vi "run.vi"() -> ()   [LabVIEW 2017]
uses:
  <vilib>/Instr/_visa.llb/VISA Configure Serial Port (Instr).vi
panel:
  in  "设备检查":bool
  out "预压？":bool=TRUE
  in  "精度":dbl=0.0005
  out "测试时断开电源？":bool=TRUE
  out "多通道/单通道":bool=TRUE
  out "压力点个数":i32
  in  "退出":bool
  out "组装调试":bool=TRUE
  in  "控制板":refnum<visa-resource-name>="COM16"
  in  "时漂测试间隔时间(min)":i32=30
  in  "时漂测试":bool
  out "时漂":dbl
  out "时漂测试数据":i32[](listbox)
  out "时漂常压输出":string[][](array[string])
  out "错误输出 3":errorcluster caption="错误输出"
  in  "温度显示编号":enum16{""}(ring)
  out "曲线拟合参数":string
  in  "传感器显示编号":u16(ring) items=["1", "2", "3", "4", "5", "6", "7", "8", "9"]
  out "显示数据":i32[](listbox)
  out "XY图":cluster{i32[], i32[]}[](graph)
  out "结束":bool
  out "显示数据":string[][](array[string])
  out "数据":string[][](array[string])
  out "错误输出 2":errorcluster caption="错误输出"
  out "压力稳定":bool
  out "压力最小值":dbl
  out "压力最大值":dbl
  out "保存名":string
  out "path":string
  out "错误输出":errorcluster
  out "恒温结束时间":string
  out "恒温开始时间":string
  out "恒温结束分钟":i32
  out "恒温结束小时":i32
  out "分钟":i32
  out "小时":i32
  out "开始上电":bool
  out "恒温开始":bool
  out "开始采集":bool
  out "传感器预热":bool
  out "恒温中":bool
  out "温度校验次数":dbl
  out "实时压力kPa":string
  out "实时温度℃":dbl
  out "当前设定温度℃":dbl
  out "温度点":i32
  in  "温度（℃）":dbl[](array[numeric])=[25.0]
  in  "CONST820":refnum<visa-resource-name>="COM3"
  in  "传感器顺序编号（从1开始）":string[](array[string])=["1", "2", "3", "4", "5", "6", "7", "8", "9"]
  in  "第二路电流 （A）":dbl=1.0
  in  "第二路电压（V）":dbl=5.0
  in  "第一路电压（V）":dbl=15.0
  in  "第一路电流（A）":dbl=1.0
  in  "DH1766-2":refnum<visa-resource-name>="COM5"
  in  "检定次数":i32=1
  in  "恒温时间（分钟）":i32=60
  in  "传感器预热时间（分钟）":i32=30
  in  "GWS":refnum<visa-resource-name>="COM4"
  in  "温度上限（℃）":dbl=75.0
  in  "温度下限（℃）":dbl=-45.0
  in  "HP34401":refnum<visa-resource-name>="COM1"
  in  "压力设定值（KPa）":dbl[](array[numeric])=[100.0, 15000.0]
  in  "STOP":bool
  out "loging":string
  out "GWS":bool
  in  "START":bool
  # "多通道 传感器测试系统"
  # "注意：\n系统测试与调试被整体集成在一起，可在主界面统一调用该页面。该页面执行完成后，返回主页面进行参数计算。\n温度设置：如需要进行自动 参数计算，请设置20℃附近常温。如不需要请忽略。\n传感器编号请从1开始，逐加。\n如需进行时漂测试，请只设置常温常压。\n\n调试测试时分两步进行：\n1、补偿电阻计算测试：\n温度设置-40℃，70℃。压力设置20KPa,15000KPa.\n2、偏置增益计算测试：\n温度设置20℃。压力设置20KPa, 100KPa, 1000KPa, 5000KPa, 10000KPa, 15000KPa。\n\n系统测试时：\n温度设置20℃， 压力设置20KPa, 100KPa, 1000KPa, 5000KPa, 10000KPa, 15000KPa。\n\n温漂测试时：\n温度设置20℃， 压力设置100KPa"
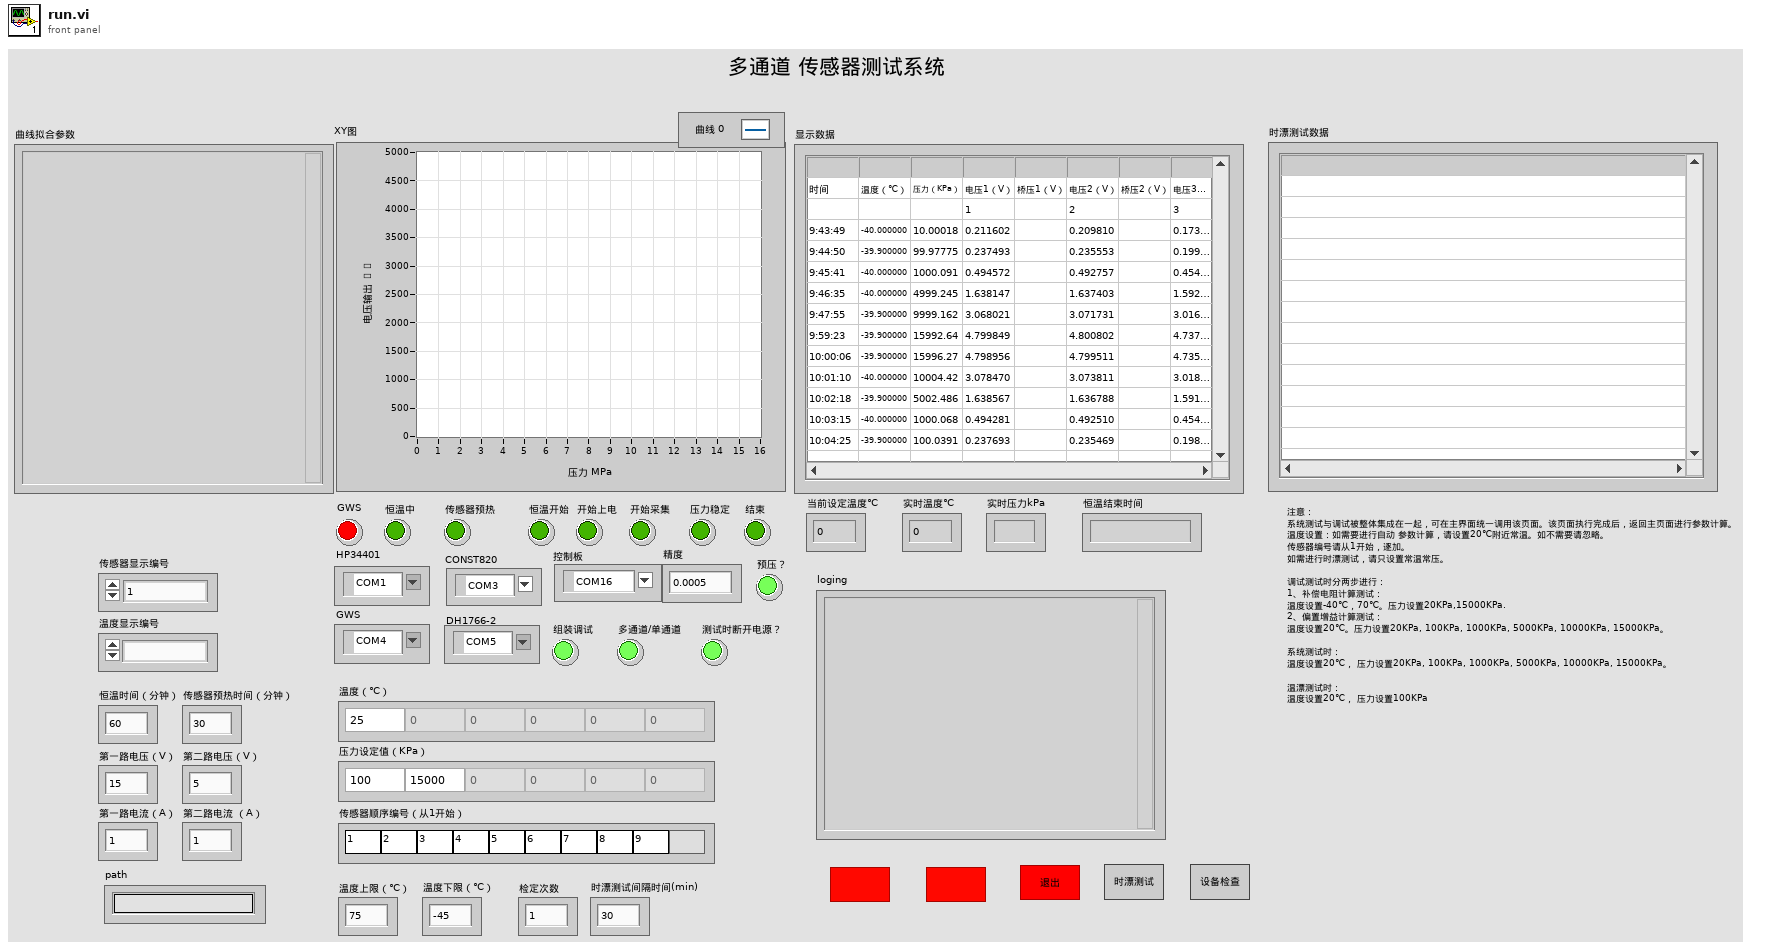
[diagram p1: front panel]
types:
  T1 = enum8{"Enabled", "Disabled", "Disabled and Grayed Out"}
  T2 = enum16{"open", "open or create", "create or replace", "create", "open (read-only)"}
  T3 = enum32{"Invalid", "Standard", "Closed", "Hidden", "Minimized", "Maximized"}
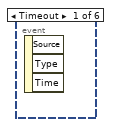
[diagram p2: hidden frame]
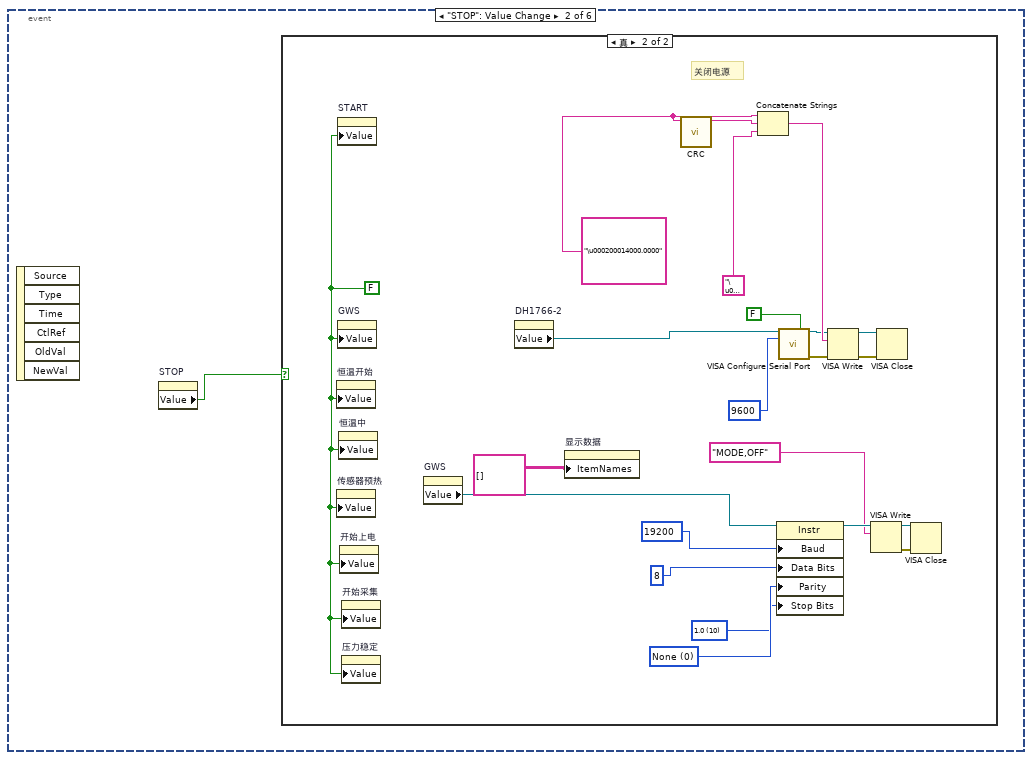
[diagram p3: hidden frame]
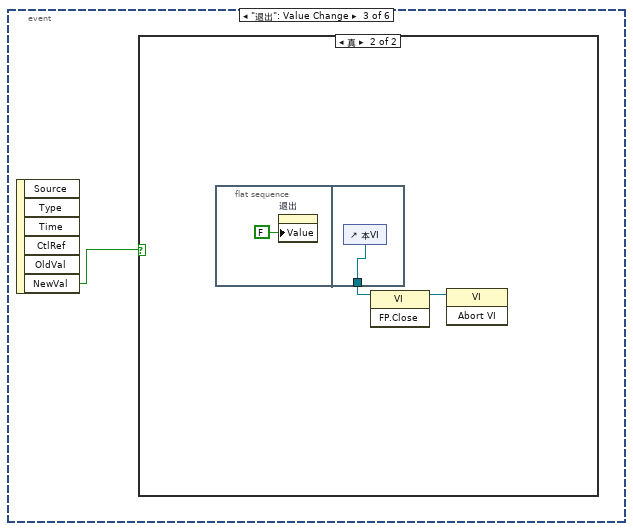
[diagram p5: hidden frame]
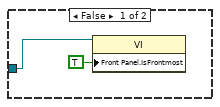
[diagram p8: hidden frame]
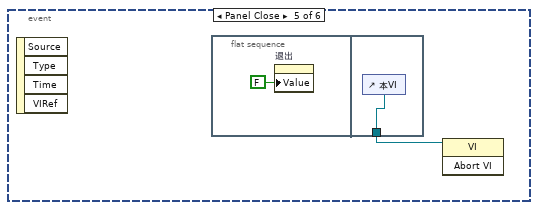
[diagram p9: hidden frame]
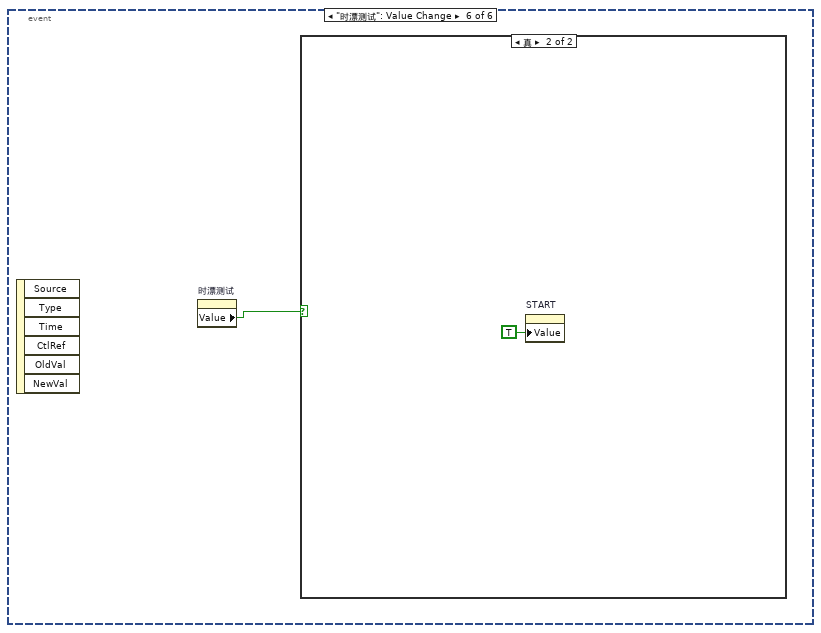
[diagram p10: hidden frame]
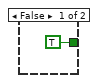
[diagram p14: hidden frame]
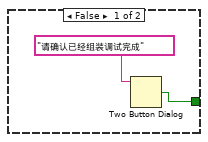
[diagram p15: hidden frame]
diagram:
  n1 = flat-sequence {
    frame #0 {
      w4 = FALSE ("恒温开始")
      w3 = FALSE ("参数计算")
      w5 = string[][] []
      w10 = ""
      w11 = 0.0
      w2 = FALSE
      # "时漂测试开始不用规定"
      n2 = disable-structure shown="禁用" {
        frame Disabled {
          n3 = property on="检定次数" class="DigNum (严格)" props=["Value"]() -> ()  [unwired: 3 in, 2 out]
        }
        frame Enabled {
        }
      }
      n4 = property on="START" class="Bool (严格)"("Value"=w2) -> ()  [unwired: 2 in, 2 out]
      n5 = property on="STOP" class="Bool (严格)"("Value"=w2) -> ()  [unwired: 2 in, 2 out]
      n6 = property on="设备检查" class="Bool (严格)"("Value"=w2) -> ()  [unwired: 2 in, 2 out]
      n7 = property on="显示数据" class="MCListbox (严格)"("ItemNames"=w5) -> ()  [unwired: 2 in, 2 out]
      n8 = property on="时漂测试数据" class="MCListbox (严格)"("ItemNames"=w5) -> ()  [unwired: 2 in, 2 out]
      n9 = property on="时漂测试" class="Bool (严格)"("Value"=w3) -> ()  [unwired: 2 in, 2 out]
      n10 = property on="时漂常压输出" class="Arr (严格)"("Value"=w5) -> ()  [unwired: 2 in, 2 out]
      n11 = property on="退出" class="Bool (严格)"("Value"=w3) -> ()  [unwired: 2 in, 2 out]
      "GWS" <- w2
      "loging" <- w10
      "温度点" <- 0 ("温度点")
      "当前设定温度℃" <- w11
      "实时温度℃" <- w11
      "实时压力kPa" <- w10
      "温度校验次数" <- 5.0 ("温度校验次数")
      "恒温开始" <- w4
      "恒温中" <- w4
      "传感器预热" <- w4
      "恒温结束时间" <- "" ("恒温结束时间")
      "开始上电" <- w4
      "开始采集" <- w4
      "压力稳定" <- w4
      "数据" <- w5
      "显示数据" <- w5
      "结束" <- w2
      "曲线拟合参数" <- "" ("曲线拟合参数")
      "时漂常压输出" <- w5
      "XY图" <- cluster{i32[], i32[]}[] []
    }
    frame #1 {
      n12 = while {
        stop <- FALSE stop-if-true
        # "start循环"
        n13 = property on="START" class="Bool (严格)"() -> ("Value"=w14:bool)  [unwired: 2 in, 2 out]
        n14 = And(x=w14, y=TRUE) -> (x .and. y?=w13:bool)
        n15 = case shown="真" w13 {
          frame False {
          }
          frame True {
            # "start点击判断"
            # "启动系统start"
            n16 = First Call?() -> (First Call?: T/F=w17:bool)
            n17 = property on="传感器预热时间（分钟）" class="DigNum (严格)"() -> ("Value"=w42:i32)  [unwired: 2 in, 2 out]
            n18 = property on="恒温时间（分钟）" class="DigNum (严格)"() -> ("Value"=w43:i32)  [unwired: 2 in, 2 out]
            n19 = property on="温度下限（℃）" class="DigNum (严格)"() -> ("Value"=w58:dbl)  [unwired: 2 in, 2 out]
            n20 = property on="温度上限（℃）" class="DigNum (严格)"() -> ("Value"=w59:dbl)  [unwired: 2 in, 2 out]
            n21 = property on="GWS" class="VISAName"() -> ("Value"=w71:refnum<visa-resource-name>)  [unwired: 2 in, 2 out]
            n22 = property on="检定次数" class="DigNum (严格)"() -> ("Value"=w40:i32)  [unwired: 2 in, 2 out]
            n23 = property on="DH1766-2" class="VISAName"() -> ("Value"=w69:refnum<visa-resource-name>)  [unwired: 2 in, 2 out]
            n24 = property on="CONST820" class="VISAName"() -> ("Value"=w67:refnum<visa-resource-name>)  [unwired: 2 in, 2 out]
            n25 = property on="HP34401" class="VISAName"() -> ("Value"=w65:refnum<visa-resource-name>)  [unwired: 2 in, 2 out]
            n26 = property on="温度（℃）" class="Arr (严格)"() -> ("Value"=w30:dbl[])  [unwired: 2 in, 2 out]
            n27 = property on="压力设定值（KPa）" class="Arr (严格)"() -> ("Value"=w35:dbl[])  [unwired: 2 in, 2 out]
            n28 = property on="传感器顺序编号（从1开始）" class="Arr (严格)"() -> ("Value"=w25:string[])  [unwired: 2 in, 2 out]
            n29 = case shown="真" w17 {
              tunnel: [TRUE ("T button?") w79] -> w16
              frame False {
              }
              frame True {
                n30 = property on="组装调试" class="Bool (严格)"() -> ("Value"=w80:bool)  [unwired: 2 in, 2 out]
                n31 = case shown="真" w80 {
                  tunnel: [w81 w83] -> w79
                  frame False {
                    n32 = Two Button Dialog(message="请确认已经组装调试完成" ("消息")) -> (T button?=w81:bool)  [unwired: 2 in]
                  }
                  frame True {
                    n33 = Two Button Dialog(message="请确认进行组装调试" ("消息")) -> (T button?=w83:bool)  [unwired: 2 in]
                  }
                }
              }
            }
            n34 = Greater Than 0?(x=w40) -> (x > 0?=w39:bool)
            n35 = Greater Than 0?(x=w42) -> (x > 0?=w54:bool)
            n36 = Greater Than 0?(x=w43) -> (x > 0?=w44:bool)
            n37 = Greater Or Equal?(x=w43, y=w42) -> (x >= y?=w41:bool)
            n38 = Array Size(array=w30) -> (size(s)=w29:i32)
            n39 = Array Size(array=w35) -> (size(s)=w33:i32)
            n40 = String Length(string=w71) -> (length=w70:i32)
            n41 = Array Size(array=w25) -> (size(s)=w24:i32)
            n42 = String Length(string=w69) -> (length=w68:i32)
            n43 = String Length(string=w67) -> (length=w66:i32)
            n44 = String Length(string=w65) -> (length=w64:i32)
            n45 = Less Or Equal To 0?(x=w29) -> (x <= 0?=w27:bool)
            n46 = Less Or Equal To 0?(x=w33) -> (x <= 0?=w32:bool)
            n47 = Greater Or Equal?(x=w59, y=w58) -> (x >= y?=w57:bool)
            n48 = Less Or Equal To 0?(x=w24) -> (x <= 0?=w23:bool)
            n49 = Equal?(x=w70, y=0) -> (x = y?=w73:bool)
            n50 = Equal?(x=w68, y=0) -> (x = y?=w72:bool)
            n51 = Equal?(x=w66, y=0) -> (x = y?=w75:bool)
            n52 = Equal?(x=w64, y=0) -> (x = y?=w76:bool)
            n53 = case shown="假" w57 {
              tunnel: ["温度上限>=温度下限 \n" _] -> w51
              frame False {
              }
              frame True {
              }
            }
            n54 = And(x=w44, y=w54) -> (x .and. y?=w38:bool)
            n55 = And(x=w39, y=w38) -> (x .and. y?=w37:bool)
            n56 = And(x=w37, y=w41) -> (x .and. y?=w36:bool)
            n57 = case shown="真" w27 {
              tunnel: [_ "请设置温度\n"] -> w28
              frame False {
              }
              frame True {
              }
            }
            n58 = case shown="真" w32 {
              tunnel: [_ "请设置压力\n"] -> w34
              frame False {
              }
              frame True {
              }
            }
            n59 = case shown="真" w23 {
              tunnel: [_ "请设置传感器编号\n"] -> w21
              frame False {
              }
              frame True {
              }
            }
            n60 = Not(x=w57) -> (.not. x?=w55:bool)
            n61 = Or(x=w72, y=w73) -> (x .or. y?=w74:bool)
            n62 = Or(x=w75, y=w74) -> (x .or. y?=w77:bool)
            n63 = Or(x=w76, y=w77) -> (x .or. y?=w56:bool)
            n64 = Not(x=w36) -> (.not. x?=w52:bool)
            n65 = case shown="假" w36 {
              tunnel: ["检定次数、恒温时间、传感器预热时间均应大于0、恒温时间>=传感器预热时间 " _] -> w47
              frame False {
              }
              frame True {
              }
            }
            n66 = Or(x=w56, y=w55) -> (x .or. y?=w53:bool)
            n67 = case shown="真" w56 {
              tunnel: [_ "部分资源未引用 "] -> w48
              frame False {
              }
              frame True {
              }
            }
            n68 = Not(x=w16) -> (.not. x?=w18:bool)
            n69 = Or(x=w53, y=w52) -> (x .or. y?=w31:bool)
            n70 = Or(x=w31, y=w32) -> (x .or. y?=w26:bool)
            n71 = Or(x=w26, y=w27) -> (x .or. y?=w22:bool)
            n72 = Or(x=w22, y=w23) -> (x .or. y?=w20:bool)
            n73 = Or(x=w20, y=w18) -> (x .or. y?=w19:bool)
            n74 = Concatenate Strings(w48, w51, w47, w34, w28, w21) -> (w45:string)
            n75 = Search and Replace String(input string=w45, search string=" " ("搜索字符串"), replace string="\r") -> (result string=w49:string)  [unwired: 5 in, 3 out]
            n76 = case shown="假" w19 {
              tunnel: w49 -> [_ w950]
              frame False {
                n77 = First Call?() -> (First Call?: T/F=w90:bool)
                n78 = case shown="真" w90 {
                  frame False {
                  }
                  frame True {
                    n79 = property on="传感器顺序编号（从1开始）" class="Arr (严格)"() -> ("Value"=w96:string[])  [unwired: 2 in, 2 out]
                    n80 = property on="时漂测试" class="Bool (严格)"() -> ("Value"=w101:bool)  [unwired: 2 in, 2 out]
                    n81 = disable-structure shown="禁用" {
                      frame Disabled {
                        n82 = property on="温度（℃）" class="Arr (严格)"() -> ("Value"=w107:dbl[])  [unwired: 2 in, 2 out]
                        n83 = Sort 1D Array(array=w107) -> (sorted array=w108:dbl[])
                        n84 = property on="温度（℃）" class="Arr (严格)"("Value"=w108) -> ()  [unwired: 2 in, 2 out]
                      }
                      frame Enabled {
                      }
                    }
                    n85 = property on="压力设定值（KPa）" class="Arr (严格)"() -> ("Value"=w95:dbl[])  [unwired: 2 in, 2 out]
                    n86 = for {
                      tunnel: w96 -> [w118] mode=indexing
                      shift-right: [w120] -> w93
                      shift-left: string[] [] -> [w119]
                      n87 = call <vilib>:"Trim Whitespace.vi"("string"=w118) -> ("trimmed string"=w117:string)  [unwired: 1 in]
                      n88 = String Length(string=w117) -> (length=w122:i32)
                      n89 = Equal To 0?(x=w122) -> (x = 0?=w121:bool)
                      n90 = case shown="真" w121 {
                        tunnel: w117 -> [w125 _]
                        tunnel: [w124 w126] -> w120
                        tunnel: w119 -> [w123 w128]
                        frame False {
                          n91 = Build Array (concatenate)(w123, w125) -> (w124:string[])
                        }
                        frame True {
                          n92 = Insert Into Array(array=w128, new element=string[] []) -> (w126:string[])  [unwired: 1 in]
                        }
                      }
                    }
                    n93 = property on="恒温时间（分钟）" class="DigNum (严格)"() -> ("Value"=w104:i32)  [unwired: 2 in, 2 out]
                    n94 = property on="时漂测试间隔时间(min)" class="DigNum (严格)"() -> ("Value"=w102:i32)  [unwired: 2 in, 2 out]
                    n95 = for {
                      tunnel: w95 -> [w109] mode=indexing
                      shift-right: [w112] -> w94
                      shift-left: dbl[] [] -> [w111]
                      n96 = Less Or Equal To 0?(x=w109) -> (x <= 0?=w110:bool)
                      n97 = case shown="假" w110 {
                        tunnel: [w115 w116] -> w112
                        tunnel: w111 -> [w114 w116]
                        tunnel: w109 -> [w113 _]
                        frame False {
                          n98 = Build Array (concatenate)(w114, w113) -> (w115:dbl[])
                        }
                        frame True {
                        }
                      }
                    }
                    n99 = Multiply(x=w102, y=8) -> (x*y=w103:i32)
                    n100 = Add(x=w103, y=w104) -> (x+y=w105:i32)
                    n101 = Number To Decimal String(number=w105) -> (decimal integer string=w106:string)  [unwired: 1 in]
                    n102 = case shown="真" w101 {
                      tunnel: w106 -> [_ w131]
                      frame False {
                      }
                      frame True {
                        n103 = Concatenate Strings("计算时间漂移、大约用时：" ("字符串"), w131, " min", "\n") -> (w133:string)
                        n104 = property on="loging" class="Str"("Value"=w133) -> ()  [unwired: 2 in, 2 out]
                      }
                    }
                    n105 = property on="压力设定值（KPa）" class="Arr (严格)"("Value"=w94) -> ()  [unwired: 2 in, 2 out]
                    n106 = Array Size(array=w94) -> (size(s)=w97:i32)
                    n107 = property on="传感器顺序编号（从1开始）" class="Arr (严格)"("Value"=w93) -> ()  [unwired: 2 in, 2 out]
                    n108 = property on="检定次数" class="DigNum (严格)"("DisabledEnum"=T1."Enabled" ("禁用")) -> ()  [unwired: 2 in, 2 out]
                    n109 = property on="压力点个数" class="DigNum (严格)"("Value"=w97) -> ()  [unwired: 2 in, 2 out]
                    n110 = property on="结束" class="Bool (严格)"("Value"=FALSE ("结束")) -> ()  [unwired: 2 in, 2 out]
                    n111 = property on="传感器显示编号" class="Ring (严格)"("Strings []"=w93) -> ()  [unwired: 2 in, 2 out]
                  }
                }
                n112 = flat-sequence {
                  frame #0 {
                    # "设置正确"
                    # "启动温箱"
                    n113 = property on="GWS" class="Bool (严格)"() -> ("Value"=w134:bool)  [unwired: 2 in, 2 out]
                    n114 = case shown="假" w134 {
                      frame False {
                        n115 = flat-sequence {
                          tunnel: [w160] -> w140
                          tunnel: [w159] -> w139
                          tunnel: [w183] -> w142
                          tunnel: [w182] -> w141
                          tunnel: w140 -> [w180]
                          tunnel: w139 -> [w179]
                          tunnel: [w199] -> w152
                          tunnel: w142 -> [w199]
                          tunnel: [w198] -> w151
                          tunnel: w141 -> [w198]
                          tunnel: w152 -> [w201]
                          tunnel: w151 -> [w202]
                          tunnel: [w201] -> w150
                          tunnel: [w200] -> w147
                          tunnel: w150 -> [w209]
                          tunnel: [w209] -> w149
                          tunnel: [w208] -> w148
                          tunnel: w147 -> [w208]
                          tunnel: w149 -> [w218]
                          tunnel: w148 -> [w217]
                          tunnel: [w213] -> w145
                          tunnel: [w212] -> w144
                          tunnel: [w222] -> w146
                          tunnel: w145 -> [w222]
                          tunnel: w144 -> [w221]
                          tunnel: [w221] -> w143
                          tunnel: w146 -> [w233]
                          tunnel: w143 -> [w232]
                          tunnel: [w228] -> _
                          frame #0 {
                            w164 = u16 10 items=["1.0"=10, "1.5"=15, "2.0"=20] ("stop bits (10: 1 bit)")
                            n116 = property on="GWS" class="VISAName"() -> ("Value"=w163:refnum<visa-resource-name>)  [unwired: 2 in, 2 out]
                            n117 = property on="loging" class="Str"() -> ("Value"=w156:string)  [unwired: 2 in, 2 out]
                            n118 = Concatenate Strings(w156, "\n启动温箱" ("字符串"), "\n") -> (w155:string)
                            n119 = call-poly "VISA Configure Serial Port"("VISA resource name"=w163, "baud rate (9600)"=u32 19200, "data bits (8)"=u16 8, "parity (0:none)"=enum16{"None", "Odd", "Even", "Mark", "Space"}."None", "stop bits (10: 1 bit)"=w164) -> ("VISA resource name out"=w158:refnum<visa-resource-name>, "error out"=w162:errorcluster)  [unwired: 9 in]
                            n120 = flat-sequence {
                              tunnel: w162 -> [w169]
                              tunnel: [w169] -> w161
                              tunnel: w158 -> [w168]
                              tunnel: [w168] -> w157
                              frame #0 {
                                n121 = Wait (ms)(milliseconds to wait=u32 20 ("等待时间（毫秒）")) -> ()  [unwired: 1 out]
                              }
                            }
                            n122 = property on="loging" class="Str"("Value"=w155) -> ()  [unwired: 2 in, 2 out]
                            n123 = VISA Open(error in (no error)=w161, VISA resource name=w157) -> (VISA resource name=w160:refnum<visa-resource-name>, error out=w159:errorcluster)  [unwired: 3 in]
                          }
                          frame #1 {
                            w187 = i16 1 ("精度(6)")
                            n124 = property on="时漂测试" class="Bool (严格)"() -> ("Value"=w171:bool)  [unwired: 2 in, 2 out]
                            n125 = property on="loging" class="Str"() -> ("Value"=w178:string)  [unwired: 2 in, 2 out]
                            n126 = property on="温度下限（℃）" class="DigNum (严格)"() -> ("Value"=w189:dbl)  [unwired: 2 in, 2 out]
                            n127 = property on="温度上限（℃）" class="DigNum (严格)"() -> ("Value"=w188:dbl)  [unwired: 2 in, 2 out]
                            n128 = case shown="假" w171 {
                              tunnel: [w193 20.0] -> w172
                              frame False {
                                n129 = property on="温度（℃）" class="Arr (严格)"() -> ("Value"=w195:dbl[])  [unwired: 2 in, 2 out]
                                n130 = property on="温度点" class="DigNum (严格)"() -> ("Value"=w194:i32)  [unwired: 2 in, 2 out]
                                n131 = Index Array(array=w195, index=w194) -> (element=w193:dbl)
                                n132 = property on="当前设定温度℃" class="DigNum (严格)"("Value"=w193) -> ()  [unwired: 2 in, 2 out]
                              }
                              frame True {
                              }
                            }
                            n133 = Number To Fractional String(number=w172, precision (6)=i16 2 ("精度(6)")) -> (F-format string=w174:string)  [unwired: 2 in]
                            n134 = Concatenate Strings(w178, "设定温度 " ("字符串"), w174, "\n") -> (w175:string)
                            n135 = Number To Fractional String(number=w172, precision (6)=w187) -> (F-format string=w192:string)  [unwired: 2 in]
                            n136 = Number To Fractional String(number=w188, precision (6)=w187) -> (F-format string=w190:string)  [unwired: 2 in]
                            n137 = Number To Fractional String(number=w189, precision (6)=w187) -> (F-format string=w191:string)  [unwired: 2 in]
                            n138 = property on="loging" class="Str"("Value"=w175) -> ()  [unwired: 2 in, 2 out]
                            n139 = Concatenate Strings("TEMP,S" ("字符串"), w192, " H" ("字符串"), w190, " L" ("字符串"), w191) -> (w181:string)
                            n140 = VISA Write(VISA resource name=w180, write buffer=w181, error in (no error)=w179) -> (VISA resource name out=w183:refnum<visa-resource-name>, error out=w182:errorcluster)  [unwired: 1 out]
                          }
                          frame #2 {
                            n141 = Wait (ms)(milliseconds to wait=u32 100 ("等待时间（毫秒）")) -> ()  [unwired: 1 out]
                          }
                          frame #3 {
                            n142 = Get Date/Time In Seconds() -> (seconds since 1Jan1904=w205:timestamp)
                            n143 = Get Date/Time String(seconds (now)=w205, want seconds? (F)=TRUE ("需要秒？(F)")) -> (time string=w207:string)  [unwired: 1 in, 1 out]
                            n144 = Concatenate Strings("TIME, " ("字符串"), w207) -> (w203:string)
                            n145 = VISA Write(VISA resource name=w201, write buffer=w203, error in (no error)=w202) -> (error out=w200:errorcluster)  [unwired: 2 out]
                          }
                          frame #4 {
                            n146 = Wait (ms)(milliseconds to wait=u32 100 ("等待时间（毫秒）")) -> ()  [unwired: 1 out]
                          }
                          frame #5 {
                            n147 = VISA Write(VISA resource name=w218, write buffer="TEMP？" ("写入缓冲区"), error in (no error)=w217) -> (VISA resource name out=w219:refnum<visa-resource-name>, error out=w214:errorcluster)  [unwired: 1 out]
                            n148 = property class="Instr"(reference=w219, error in=w214) -> (reference out=w216:refnum<visa-resource-name>, error out=w211:errorcluster, "Bytes at Port"=w215:u32)
                            n149 = VISA Read(VISA resource name=w216, byte count=w215, error in (no error)=w211) -> (VISA resource name out=w213:refnum<visa-resource-name>, error out=w212:errorcluster)  [unwired: 2 out]
                          }
                          frame #6 {
                            n150 = Wait (ms)(milliseconds to wait=u32 100 ("等待时间（毫秒）")) -> ()  [unwired: 1 out]
                          }
                          frame #7 {
                            n151 = property on="loging" class="Str"() -> ("Value"=w227:string)  [unwired: 2 in, 2 out]
                            n152 = Concatenate Strings(w227, "温箱已启动" ("字符串"), "\n") -> (w225:string)
                            n153 = property on="GWS" class="Bool (严格)"("Value"=TRUE ("GWS")) -> ()  [unwired: 2 in, 2 out]
                            n154 = VISA Write(VISA resource name=w233, write buffer="MODE,CONSTANT" ("写入缓冲区"), error in (no error)=w232) -> (VISA resource name out=w230:refnum<visa-resource-name>, error out=w229:errorcluster)  [unwired: 1 out]
                            n155 = property on="loging" class="Str"("Value"=w225) -> ()  [unwired: 2 in, 2 out]
                            n156 = VISA Close(VISA resource name=w230, error in (no error)=w229) -> (error out=w228:errorcluster)
                          }
                        }
                      }
                      frame True {
                      }
                    }
                    n157 = disable-structure shown="禁用" {
                      frame Disabled {
                        n158 = property on="loging" class="Str"() -> ("Value"=w137:string)  [unwired: 2 in, 2 out]
                        n159 = Concatenate Strings(w137, "温箱已启动" ("字符串"), "\n") -> (w138:string)
                        n160 = property on="loging" class="Str"("Value"=w138) -> ()  [unwired: 2 in, 2 out]
                      }
                      frame Enabled {
                      }
                    }
                  }
                  frame #1 {
                    # "温箱温度检查"
                    n161 = property on="温度校验次数" class="DigNum (严格)"() -> ("Value"=w236:dbl)  [unwired: 2 in, 2 out]
                    n162 = disable-structure shown="禁用" {
                      frame Disabled {
                        n163 = property on="温度校验次数" class="DigNum (严格)"() -> ("Value"=w238:dbl)  [unwired: 2 in, 2 out]
                        n164 = Greater Than 0?(x=w238) -> (x > 0?=w237:bool)
                        n165 = case shown="真" w237 {
                          frame False {
                          }
                          frame True {
                            n166 = property on="loging" class="Str"() -> ("Value"=w241:string)  [unwired: 2 in, 2 out]
                            n167 = Concatenate Strings(w241, "温箱温度监控" ("字符串"), "\n") -> (w242:string)
                            n168 = property on="loging" class="Str"("Value"=w242) -> ()  [unwired: 2 in, 2 out]
                          }
                        }
                      }
                      frame Enabled {
                      }
                    }
                    n169 = Greater Than 0?(x=w236) -> (x > 0?=w235:bool)
                    n170 = case shown="真" w235 {
                      frame False {
                      }
                      frame True {
                        n171 = while {
                          stop <- w247 stop-if-true
                          n172 = flat-sequence {
                            tunnel: [w254] -> w252
                            tunnel: [w253] -> w251
                            tunnel: [w261] -> w250
                            tunnel: w252 -> [w261]
                            tunnel: [w260] -> w249
                            tunnel: w251 -> [w260]
                            tunnel: w250 -> [w271]
                            tunnel: w249 -> [w270]
                            frame #0 {
                              n173 = property on="GWS" class="VISAName"() -> (error out=w258:errorcluster, "Value"=w259:refnum<visa-resource-name>)  [unwired: 2 in, 1 out]
                              n174 = VISA Flush I/O Buffer(VISA resource name=w259, error in (no error)=w258) -> (VISA resource name out=w256:refnum<visa-resource-name>, error out=w257:errorcluster)  [unwired: 1 in]
                              n175 = VISA Write(VISA resource name=w256, write buffer="TEMP?" ("写入缓冲区"), error in (no error)=w257) -> (VISA resource name out=w254:refnum<visa-resource-name>, error out=w253:errorcluster)  [unwired: 1 out]
                            }
                            frame #1 {
                              n176 = Wait (ms)(milliseconds to wait=u32 100 ("等待时间（毫秒）")) -> ()  [unwired: 1 out]
                            }
                            frame #2 {
                              n177 = property class="Instr"(reference=w271, error in=w270) -> (reference out=w269:refnum<visa-resource-name>, error out=w267:errorcluster, "Bytes at Port"=w268:u32)
                              n178 = VISA Read(VISA resource name=w269, byte count=w268, error in (no error)=w267) -> (read buffer=w264:string)  [unwired: 3 out]
                              n179 = Match Pattern(string=w264, regular expression="," ("正则表达式")) -> (before substring=w263:string)  [unwired: 1 in, 3 out]
                              n180 = Fract/Exp String To Number(string=w263) -> (number=w266:dbl)  [unwired: 3 in, 1 out]
                              n181 = property on="实时温度℃" class="DigNum (严格)"("Value"=w266) -> ()  [unwired: 2 in, 2 out]
                            }
                            frame #3 {
                              n182 = Wait (ms)(milliseconds to wait=u32 100 ("等待时间（毫秒）")) -> ()  [unwired: 1 out]
                            }
                            frame #4 {
                              w279 = 0.1 ("y")
                              n183 = property on="当前设定温度℃" class="DigNum (严格)"() -> ("Value"=w280:dbl)  [unwired: 2 in, 2 out]
                              n184 = property on="实时温度℃" class="DigNum (严格)"() -> ("Value"=w275:dbl)  [unwired: 2 in, 2 out]
                              n185 = Add(x=w280, y=w279) -> (x+y=w274:dbl)
                              n186 = Greater Or Equal?(x=w274, y=w275) -> (x >= y?=w278:bool)
                              n187 = Subtract(x=w280, y=w279) -> (x-y=w273:dbl)
                              n188 = Greater Or Equal?(x=w275, y=w273) -> (x >= y?=w277:bool)
                              n189 = And(x=w278, y=w277) -> (x .and. y?=w276:bool)
                              n190 = In Range and Coerce(upper limit=w274, x=w275, lower limit=w273) -> ()  [unwired: 2 out]
                              n191 = case shown="真" w276 {
                                frame False {
                                }
                                frame True {
                                n192 = property on="温度校验次数" class="DigNum (严格)"() -> ("Value"=w281:dbl)  [unwired: 2 in, 2 out]
                                n193 = Less Or Equal To 0?(x=w281) -> (x <= 0?=w282:bool)
                                n194 = Decrement(x=w281) -> (x-1=w283:dbl)
                                n195 = case shown="真" w282 {
                                frame False {
                                }
                                frame True {
                                n196 = property on="恒温开始" class="Bool (严格)"("Value"=TRUE ("恒温开始")) -> ()  [unwired: 2 in, 2 out]
                                }
                                }
                                n197 = property on="温度校验次数" class="DigNum (严格)"("Value"=w283) -> ()  [unwired: 2 in, 2 out]
                                }
                              }
                            }
                          }
                          n198 = property on="温度校验次数" class="DigNum (严格)"() -> ("Value"=w248:dbl)  [unwired: 2 in, 2 out]
                          n199 = Less Or Equal To 0?(x=w248) -> (x <= 0?=w247:bool)
                        }
                        n200 = property on="loging" class="Str"() -> ("Value"=w246:string)  [unwired: 2 in, 2 out]
                        n201 = Concatenate Strings(w246, "温箱温度监控、恒温检查中" ("字符串"), "\n") -> (w244:string)
                        n202 = property on="loging" class="Str"("Value"=w244) -> ()  [unwired: 2 in, 2 out]
                      }
                    }
                  }
                  frame #2 {
                    # "恒温到达时间计算"
                    n203 = property on="恒温开始" class="Bool (严格)"() -> ("Value"=w285:bool)  [unwired: 2 in, 2 out]
                    n204 = case shown="真" w285 {
                      frame False {
                      }
                      frame True {
                        w295 = TRUE ("恒温中")
                        n205 = Get Date/Time In Seconds() -> (seconds since 1Jan1904=w309:timestamp)
                        n206 = property on="loging" class="Str"() -> ("Value"=w293:string)  [unwired: 2 in, 2 out]
                        n207 = Get Date/Time String(seconds (now)=w309) -> (date string=w288:string, time string=w286:string)  [unwired: 2 in]
                        n208 = property on="恒温中" class="Bool (严格)"("Value"=w295) -> ()  [unwired: 2 in, 2 out]
                        n209 = Concatenate Strings(w293, "开始恒温，计算恒温时间" ("字符串"), "\n") -> (w290:string)
                        n210 = Concatenate Strings(w288, " " ("字符串"), w286) -> (w289:string)
                        n211 = Match Pattern(string=w286, regular expression=":" ("正则表达式")) -> (before substring=w308:string, after substring=w307:string)  [unwired: 1 in, 2 out]
                        n212 = property on="恒温开始时间" class="Str"("Value"=w289) -> ()  [unwired: 2 in, 2 out]
                        n213 = property on="loging" class="Str"("Value"=w290) -> ()  [unwired: 2 in, 2 out]
                        n214 = property on="恒温开始" class="Bool (严格)"("Value"=FALSE ("恒温开始")) -> ()  [unwired: 2 in, 2 out]
                        n215 = property on="传感器预热" class="Bool (严格)"("Value"=w295) -> ()  [unwired: 2 in, 2 out]
                        n216 = Decimal String To Number(string=w308) -> (number=w301:i32)  [unwired: 2 in, 1 out]
                        n217 = Decimal String To Number(string=w307) -> (number=w300:i32)  [unwired: 2 in, 1 out]
                        n218 = property on="分钟" class="DigNum (严格)"("Value"=w300) -> ()  [unwired: 2 in, 2 out]
                        n219 = property on="小时" class="DigNum (严格)"("Value"=w301) -> ()  [unwired: 2 in, 2 out]
                        n220 = property on="恒温时间（分钟）" class="DigNum (严格)"() -> ("Value"=w299:i32)  [unwired: 2 in, 2 out]
                        n221 = call "cal_end_time.vi"("恒温时间"=w299, "分钟"=w300, "小时"=w301) -> ("结束分钟"=w297:i32, "结束小时"=w298:i32)  [unwired: 7 in]
                        n222 = Number To Decimal String(number=w298, width (-)=i16 2 ("宽度(-)")) -> (decimal integer string=w304:string)
                        n223 = Number To Decimal String(number=w297) -> (decimal integer string=w303:string)  [unwired: 1 in]
                        n224 = Concatenate Strings(w304, ":", w303) -> (w296:string)
                        n225 = property on="恒温结束小时" class="DigNum (严格)"("Value"=w298) -> ()  [unwired: 2 in, 2 out]
                        n226 = property on="恒温结束分钟" class="DigNum (严格)"("Value"=w297) -> ()  [unwired: 2 in, 2 out]
                        n227 = property on="恒温结束时间" class="Str"("Value"=w296) -> ()  [unwired: 2 in, 2 out]
                      }
                    }
                  }
                  frame #3 {
                    # "恒温时间到达"
                    n228 = property on="恒温中" class="Bool (严格)"() -> ("Value"=w311:bool)  [unwired: 2 in, 2 out]
                    n229 = property on="传感器预热" class="Bool (严格)"() -> ("Value"=w310:bool)  [unwired: 2 in, 2 out]
                    n230 = disable-structure shown="禁用" {
                      frame Disabled {
                        n231 = property on="loging" class="Str"() -> ("Value"=w314:string)  [unwired: 2 in, 2 out]
                        n232 = Concatenate Strings(w314, "传感器预热" ("字符串"), "\n") -> (w315:string)
                        n233 = property on="loging" class="Str"("Value"=w315) -> ()  [unwired: 2 in, 2 out]
                      }
                      frame Enabled {
                      }
                    }
                    n234 = case shown="真" w311 {
                      frame False {
                      }
                      frame True {
                        n235 = Get Date/Time In Seconds() -> (seconds since 1Jan1904=w346:timestamp)
                        n236 = Get Date/Time String(seconds (now)=w346) -> (time string=w342:string)  [unwired: 2 in, 1 out]
                        n237 = property on="恒温结束分钟" class="DigNum (严格)"() -> ("Value"=w340:i32)  [unwired: 2 in, 2 out]
                        n238 = property on="恒温结束小时" class="DigNum (严格)"() -> ("Value"=w338:i32)  [unwired: 2 in, 2 out]
                        n239 = Match Pattern(string=w342, regular expression=":" ("正则表达式")) -> (before substring=w345:string, after substring=w344:string)  [unwired: 1 in, 2 out]
                        n240 = Decimal String To Number(string=w345) -> (number=w339:i32)  [unwired: 2 in, 1 out]
                        n241 = Decimal String To Number(string=w344) -> (number=w341:i32)  [unwired: 2 in, 1 out]
                        n242 = Equal?(x=w341, y=w340) -> (x = y?=w337:bool)
                        n243 = Equal?(x=w339, y=w338) -> (x = y?=w336:bool)
                        n244 = And(x=w337, y=w336) -> (x .and. y?=w335:bool)
                        n245 = case shown="真" w335 {
                          frame False {
                          }
                          frame True {
                            n246 = property on="loging" class="Str"() -> ("Value"=w351:string)  [unwired: 2 in, 2 out]
                            n247 = property on="开始采集" class="Bool (严格)"("Value"=TRUE ("开始采集")) -> ()  [unwired: 2 in, 2 out]
                            n248 = property on="恒温中" class="Bool (严格)"("Value"=FALSE ("恒温中")) -> ()  [unwired: 2 in, 2 out]
                            n249 = Concatenate Strings(w351, "恒温时间到" ("字符串"), "\n") -> (w348:string)
                            n250 = property on="loging" class="Str"("Value"=w348) -> ()  [unwired: 2 in, 2 out]
                          }
                        }
                      }
                    }
                    n251 = case shown="真" w310 {
                      frame False {
                      }
                      frame True {
                        n252 = property on="恒温时间（分钟）" class="DigNum (严格)"() -> ("Value"=w332:i32)  [unwired: 2 in, 2 out]
                        n253 = property on="传感器预热时间（分钟）" class="DigNum (严格)"() -> ("Value"=w331:i32)  [unwired: 2 in, 2 out]
                        n254 = property on="分钟" class="DigNum (严格)"() -> ("Value"=w329:i32)  [unwired: 2 in, 2 out]
                        n255 = property on="小时" class="DigNum (严格)"() -> ("Value"=w330:i32)  [unwired: 2 in, 2 out]
                        n256 = Get Date/Time In Seconds() -> (seconds since 1Jan1904=w327:timestamp)
                        n257 = Get Date/Time String(seconds (now)=w327) -> (time string=w323:string)  [unwired: 2 in, 1 out]
                        n258 = Subtract(x=w332, y=w331) -> (x-y=w328:i32)
                        n259 = call "cal_end_time.vi"("恒温时间"=w328, "分钟"=w329, "小时"=w330) -> ("结束分钟"=w319:i32, "结束小时"=w321:i32)  [unwired: 7 in]
                        n260 = Match Pattern(string=w323, regular expression=":" ("正则表达式")) -> (before substring=w326:string, after substring=w325:string)  [unwired: 1 in, 2 out]
                        n261 = Decimal String To Number(string=w326) -> (number=w322:i32)  [unwired: 2 in, 1 out]
                        n262 = Decimal String To Number(string=w325) -> (number=w320:i32)  [unwired: 2 in, 1 out]
                        n263 = Equal?(x=w320, y=w319) -> (x = y?=w317:bool)
                        n264 = Equal?(x=w322, y=w321) -> (x = y?=w318:bool)
                        n265 = And(x=w318, y=w317) -> (x .and. y?=w316:bool)
                        n266 = case shown="真" w316 {
                          frame False {
                          }
                          frame True {
                            n267 = property on="传感器预热" class="Bool (严格)"("Value"=FALSE ("传感器预热")) -> ()  [unwired: 2 in, 2 out]
                            n268 = property on="开始上电" class="Bool (严格)"("Value"=TRUE ("开始上电")) -> ()  [unwired: 2 in, 2 out]
                          }
                        }
                      }
                    }
                  }
                  frame #4 {
                    # "开始 设置电源的两路输出端"
                    n269 = property on="开始上电" class="Bool (严格)"() -> ("Value"=w353:bool)  [unwired: 2 in, 2 out]
                    n270 = case shown="真" w353 {
                      frame False {
                      }
                      frame True {
                        n271 = flat-sequence {
                          tunnel: [w365] -> w359
                          tunnel: [w364] -> w358
                          tunnel: w359 -> [w391]
                          tunnel: [w391] -> w357
                          tunnel: w358 -> [w390]
                          tunnel: [w389] -> w355
                          tunnel: w357 -> [w427]
                          tunnel: [w427] -> w356
                          tunnel: w355 -> [w426]
                          tunnel: [w426] -> w354
                          tunnel: w356 -> [w434]
                          tunnel: w354 -> [w433]
                          frame #0 {
                            # "查询设备是否开启的指令"
                            n272 = while {
                              tunnel: [w368] -> w365
                              tunnel: [w367] -> w364
                              stop <- w369 continue-if-true
                              n273 = property on="DH1766-2" class="VISAName"() -> ("Value"=w384:refnum<visa-resource-name>)  [unwired: 2 in, 2 out]
                              n274 = call-poly "VISA Configure Serial Port"("VISA resource name"=w384) -> ("VISA resource name out"=w381:refnum<visa-resource-name>, "error out"=w379:errorcluster)  [unwired: 13 in]
                              n275 = Concatenate Strings("\u000200018\u0004û" ("字符串"), "\u0003" ("字符串")) -> (w380:string)
                              n276 = VISA Write(VISA resource name=w381, write buffer=w380, error in (no error)=w379) -> (VISA resource name out=w378:refnum<visa-resource-name>, error out=w376:errorcluster)  [unwired: 1 out]
                              n277 = flat-sequence {
                                tunnel: w378 -> [w387]
                                tunnel: [w387] -> w377
                                tunnel: w376 -> [w386]
                                tunnel: [w386] -> w375
                                frame #0 {
                                n278 = Wait (ms)(milliseconds to wait=u32 100 ("等待时间（毫秒）")) -> ()  [unwired: 1 out]
                                }
                              }
                              n279 = property class="Instr"(reference=w377, error in=w375) -> (reference out=w372:refnum<visa-resource-name>, error out=w374:errorcluster, "Bytes at Port"=w373:u32)
                              n280 = VISA Read(VISA resource name=w372, byte count=w373, error in (no error)=w374) -> (VISA resource name out=w368:refnum<visa-resource-name>, read buffer=w371:string, error out=w367:errorcluster)  [unwired: 1 out]
                              n281 = Wait Until Next ms Multiple(millisecond multiple=u32 10 ("毫秒倍数")) -> ()  [unwired: 1 out]
                              n282 = Equal?(x=w371, y="") -> (x = y?=w369:bool)
                              n283 = case shown="真" w369 {
                                frame False {
                                }
                                frame True {
                                n284 = One Button Dialog(message="DH1766电源未开启" ("消息")) -> ()  [unwired: 1 in, 1 out]
                                }
                              }
                            }
                            n285 = property on="loging" class="Str"() -> ("Value"=w363:string)  [unwired: 2 in, 2 out]
                            n286 = Concatenate Strings(w363, "电源输出，开始上电，预热传感器" ("字符串"), "\n") -> (w360:string)
                            n287 = property on="loging" class="Str"("Value"=w360) -> ()  [unwired: 2 in, 2 out]
                          }
                          frame #1 {
                            # "顺序指令执行"
                            n288 = property on="第一路电流（A）" class="DigNum (严格)"() -> ("Value"=w398:dbl)  [unwired: 2 in, 2 out]
                            n289 = property on="第一路电压（V）" class="DigNum (严格)"() -> ("Value"=w397:dbl)  [unwired: 2 in, 2 out]
                            n290 = property on="第二路电压（V）" class="DigNum (严格)"() -> ("Value"=w395:dbl)  [unwired: 2 in, 2 out]
                            n291 = property on="第二路电流 （A）" class="DigNum (严格)"() -> ("Value"=w396:dbl)  [unwired: 2 in, 2 out]
                            n292 = Build Array(w398, w397, w396, w395) -> (w393:dbl[])
                            n293 = Array Size(array=w393) -> (size(s)=w394:i32)
                            n294 = Build Array("\u0002000000", "\u0002000010", "\u0002010000", "\u0002010010") -> (w392:string[])
                            n295 = for {
                              N: w394 -> [_]
                              tunnel: w393 -> [w407] mode=indexing
                              tunnel: w392 -> [w406] mode=indexing
                              tunnel: w391 -> [w405]
                              shift-right: [w403] -> w389
                              shift-left: w390 -> [w404]
                              n296 = flat-sequence {
                                tunnel: w407 -> [w412]
                                tunnel: w406 -> [w411]
                                tunnel: w405 -> [w410]
                                tunnel: w404 -> [w409]
                                tunnel: [w408] -> w403
                                frame #0 {
                                n297 = Number To Fractional String(number=w412, width (-)=7, precision (6)=i16 4 ("精度(6)")) -> (F-format string=w421:string)  [unwired: 1 in]
                                n298 = Search and Replace String(input string=w421, search string=" " ("搜索字符串"), replace string="0" ("子字符串(\"\")"), offset=0 ("偏移量(0)")) -> (result string=w422:string)  [unwired: 4 in, 3 out]
                                n299 = Concatenate Strings(w411, w422) -> (w416:string)
                                n300 = call "CRC.vi"("命令字符串"=w416) -> ("校验字符串"=w415:string)  [unwired: 10 in]
                                n301 = Concatenate Strings(w416, w415, "\u0003" ("字符串")) -> (w414:string)
                                n302 = VISA Write(VISA resource name=w410, write buffer=w414, error in (no error)=w409) -> (error out=w408:errorcluster)  [unwired: 2 out]
                                }
                                frame #1 {
                                n303 = Wait (ms)(milliseconds to wait=u32 100 ("等待时间（毫秒）")) -> ()  [unwired: 1 out]
                                }
                              }
                            }
                          }
                          frame #2 {
                            # "启动所有的节点预热"
                            n304 = property on="多通道/单通道" class="Bool (严格)"() -> ("Value"=w425:bool)  [unwired: 2 in, 2 out]
                            n305 = case shown="真" w425 {
                              frame False {
                              }
                              frame True {
                                n306 = property on="控制板" class="VISAName"() -> ("Value"=w430:refnum<visa-resource-name>)  [unwired: 2 in, 2 out]
                                n307 = property on="传感器顺序编号（从1开始）" class="Arr (严格)"() -> ("Value"=w429:string[])  [unwired: 2 in, 2 out]
                                n308 = Array Size(array=w429) -> (size(s)=w428:i32)
                                n309 = call "prepare_elec_sensor.vi"("传感器数目"=w428, "VISA资源名称"=w430) -> ()  [unwired: 10 in]
                              }
                            }
                          }
                          frame #3 {
                            w437 = "\u000200014111.0000"
                            # "结束配置"
                            n310 = property on="开始上电" class="Bool (严格)"("Value"=FALSE ("开始上电")) -> ()  [unwired: 2 in, 2 out]
                            n311 = call "CRC.vi"("命令字符串"=w437) -> ("校验字符串"=w438:string)  [unwired: 10 in]
                            n312 = Concatenate Strings(w437, w438, "\u0003" ("字符串")) -> (w439:string)
                            n313 = VISA Write(VISA resource name=w434, write buffer=w439, error in (no error)=w433) -> (VISA resource name out=w436:refnum<visa-resource-name>, error out=w435:errorcluster)  [unwired: 1 out]
                            n314 = VISA Close(VISA resource name=w436, error in (no error)=w435) -> (error out=→"错误输出":errorcluster)
                          }
                        }
                      }
                    }
                  }
                  frame #5 {
                    # "数值有效判断"
                    # "开始采集数据"
                    n315 = property on="开始采集" class="Bool (严格)"() -> ("Value"=w441:bool)  [unwired: 2 in, 2 out]
                    n316 = case shown="真" w441 {
                      frame False {
                      }
                      frame True {
                        n317 = flat-sequence {
                          tunnel: [w477] -> w442
                          frame #0 {
                            n318 = property on="预压？" class="Bool (严格)"() -> ("Value"=w474:bool)  [unwired: 2 in, 2 out]
                            n319 = case shown="真" w474 {
                              frame False {
                              }
                              frame True {
                                n320 = property on="压力设定值（KPa）" class="Arr (严格)"() -> ("Value"=w475:dbl[])  [unwired: 2 in, 2 out]
                                n321 = property on="CONST820" class="VISAName"() -> ("Value"=w476:refnum<visa-resource-name>)  [unwired: 2 in, 2 out]
                                n322 = call "prepare_press.vi"("压力设定值（KPa）"=w475, "CONST820"=w476) -> ()  [unwired: 10 in]
                              }
                            }
                          }
                          frame #1 {
                            n323 = property on="时漂测试" class="Bool (严格)"() -> ("Value"=w477:bool)  [unwired: 2 in, 2 out]
                          }
                        }
                        n324 = Get Date/Time String() -> (date string=w465:string, time string=w453:string)  [unwired: 3 in]
                        n325 = Search and Replace String(input string=w465, search string="/" ("搜索字符串"), replace string="" ("替换字符串(\"\")")) -> (result string=w471:string)  [unwired: 5 in, 3 out]
                        n326 = Search and Replace String(input string=w453, search string=":" ("搜索字符串"), replace string="" ("替换字符串(\"\")")) -> (result string=w457:string)  [unwired: 5 in, 3 out]
                        n327 = property on="loging" class="Str"() -> ("Value"=w463:string)  [unwired: 2 in, 2 out]
                        n328 = Search and Replace String(input string=w471, search string="/" ("搜索字符串"), replace string="" ("替换字符串(\"\")")) -> (result string=w468:string)  [unwired: 5 in, 3 out]
                        n329 = Concatenate Strings(w463, "恒温变压数据采集中" ("字符串"), "\n") -> (w460:string)
                        n330 = Search and Replace String(input string=w457, search string=":" ("搜索字符串"), replace string="" ("替换字符串(\"\")")) -> (result string=w452:string)  [unwired: 5 in, 3 out]
                        n331 = Concatenate Strings(w468, "" ("字符串")) -> (w466:string)
                        n332 = property on="loging" class="Str"("Value"=w460) -> ()  [unwired: 2 in, 2 out]
                        n333 = Concatenate Strings(w466, "_" ("字符串"), w452) -> (w449:string)
                        "保存名" <- w449
                        n334 = property on="当前设定温度℃" class="DigNum (严格)"() -> ("Value"=w464:dbl)  [unwired: 2 in, 2 out]
                        n335 = Number To Fractional String(number=w464, precision (6)=i16 1 ("精度(6)")) -> (F-format string=w447:string)  [unwired: 2 in]
                        n336 = Search and Replace String(input string=w447, search string="." ("搜索字符串"), replace string="" ("替换字符串(\"\")")) -> (result string=w444:string)  [unwired: 5 in, 3 out]
                        n337 = Concatenate Strings(w449, "_" ("字符串"), w444) -> (→"path":string)
                        n338 = case shown="真" w442 {
                          frame False {
                          }
                          frame True {
                            # "时漂执行序列"
                            # "时间漂移测试"
                            n339 = flat-sequence {
                              frame #0 {
                                n340 = for {
                                N: 9 -> [_]
                                i -> [w684]
                                # "执行序列"
                                n341 = flat-sequence {
                                tunnel: [w700] -> w695
                                tunnel: [w699] -> w689
                                tunnel: [w697] -> w685
                                tunnel: [w704] -> w696
                                tunnel: w695 -> [w704]
                                tunnel: [w703] -> w694
                                tunnel: w689 -> [w703]
                                tunnel: [w701] -> w686
                                tunnel: w685 -> [w701]
                                tunnel: w696 -> [w710]
                                tunnel: w694 -> [w709]
                                tunnel: [w708] -> w693
                                tunnel: [w707] -> w692
                                tunnel: [w706] -> w688
                                tunnel: [w705] -> w687
                                tunnel: w686 -> [w705]
                                tunnel: w693 -> [w724]
                                tunnel: w692 -> [w723]
                                tunnel: [w722] -> w691
                                tunnel: [w721] -> w690
                                tunnel: w688 -> [w720]
                                tunnel: w687 -> [w719]
                                tunnel: w691 -> [w750]
                                tunnel: w690 -> [w749]
                                tunnel: w684 -> [w838]
                                frame #0 {
                                w697 = 100.0 ("设定")
                                # "压力固定值"
                                n342 = property on="CONST820" class="VISAName"() -> ("Value"=w698:refnum<visa-resource-name>)  [unwired: 2 in, 2 out]
                                n343 = call "设定压力.vi"("设定"=w697, "VISA resource name"=w698) -> ("错误输出"=w699:errorcluster, "VISA资源名称输出"=w700:refnum<visa-resource-name>)  [unwired: 1 in]
                                }
                                frame #1 {
                                n344 = Wait (ms)(milliseconds to wait=u32 100 ("毫秒计时值")) -> ()  [unwired: 1 out]
                                }
                                frame #2 {
                                n345 = while {
                                tunnel: w710 -> [w715]
                                tunnel: w709 -> [w714]
                                tunnel: [w717] -> w706
                                tunnel: [w713] -> w708
                                tunnel: [w712] -> w707
                                stop <- w717 stop-if-true
                                # "1稳定 0不稳定"
                                n346 = call "压力稳定状态.vi"("error in (no error) 2"=w714, "VISA resource name"=w715) -> ("错误输出"=w712:errorcluster, "状态(1稳定)"=w711:string, "VISA资源名称输出"=w713:refnum<visa-resource-name>)  [unwired: 1 in]
                                n347 = Wait Until Next ms Multiple(millisecond multiple=u32 10 ("毫秒倍数")) -> ()  [unwired: 1 out]
                                n348 = Decimal String To Number(string=w711) -> (number=w718:i32)  [unwired: 2 in, 1 out]
                                n349 = Greater Than 0?(x=w718) -> (x > 0?=w717:bool)
                                }
                                n350 = property on="压力稳定" class="Bool (严格)"("Value"=w706) -> ()  [unwired: 2 in, 2 out]
                                }
                                frame #3 {
                                n351 = case shown="真" w720 {
                                tunnel: w724 -> [w726 w731]
                                tunnel: w723 -> [w725 w730]
                                tunnel: [w726 w729] -> w722
                                tunnel: [w725 w728] -> w721
                                tunnel: w719 -> [_ w727]
                                frame False {
                                }
                                frame True {
                                n352 = while {
                                tunnel: w731 -> [w741]
                                tunnel: w730 -> [w742]
                                tunnel: [w740] -> w729
                                tunnel: [w738] -> w728
                                tunnel: [w737] -> _
                                tunnel: w727 -> [w736]
                                stop <- w744 stop-if-true
                                w735 = 1.0 ("上限")
                                n353 = call "CONST820目标压力测量.vi"("error in (no error) 2"=w742, "VISA resource name"=w741) -> ("错误输出"=w738:errorcluster, "目标压力值"=w739:string, "VISA资源名称输出"=w740:refnum<visa-resource-name>)  [unwired: 1 in]
                                n354 = property on="精度" class="DigNum (严格)"() -> ("Value"=w734:dbl)  [unwired: 2 in, 2 out]
                                n355 = Wait Until Next ms Multiple(millisecond multiple=u32 10 ("毫秒倍数")) -> ()  [unwired: 1 out]
                                n356 = Add(x=w735, y=w734) -> (x+y=w733:dbl)
                                n357 = Match Pattern(string=w739, regular expression="," ("正则表达式")) -> (before substring=w737:string)  [unwired: 1 in, 3 out]
                                n358 = Subtract(x=w735, y=w734) -> (x-y=w732:dbl)
                                n359 = property on="实时压力kPa" class="Str"("Value"=w737) -> ()  [unwired: 2 in, 2 out]
                                n360 = Fract/Exp String To Number(string=w737) -> (number=w746:dbl)  [unwired: 3 in, 1 out]
                                n361 = Divide(x=w746, y=w736) -> (x/y=w745:dbl)
                                n362 = In Range and Coerce(upper limit=w733, x=w745, lower limit=w732) -> (In Range?=w744:bool)  [unwired: 1 out]
                                }
                                }
                                }
                                }
                                frame #4 {
                                n363 = VISA Close(VISA resource name=w750, error in (no error)=w749) -> (error out=→"错误输出 3":errorcluster)
                                }
                                frame #5 {
                                # "可视化"
                                # "数据采集"
                                n364 = property on="当前设定温度℃" class="DigNum (严格)"() -> ("Value"=w755:dbl)  [unwired: 2 in, 2 out]
                                n365 = property on="GWS" class="VISAName"() -> (error out=w754:errorcluster, "Value"=w753:refnum<visa-resource-name>)  [unwired: 2 in, 1 out]
                                n366 = while {
                                tunnel: w753 -> [w834]
                                tunnel: w754 -> [w833]
                                tunnel: w755 -> [w832]
                                tunnel: [w829] -> w752
                                tunnel: [w828] -> w751
                                stop <- w829 stop-if-true
                                w835 = 0.1
                                # "再次判断温度设置"
                                n367 = call "get_temp.vi"("错误输入（无错误）"=w833, "VISA资源名称"=w834) -> ("实时温度"=w828:dbl)  [unwired: 7 in, 2 out]
                                n368 = property on="实时温度℃" class="DigNum (严格)"("Value"=w828) -> ()  [unwired: 2 in, 2 out]
                                n369 = Add(x=w832, y=w835) -> (x+y=w827:dbl)
                                n370 = Subtract(x=w832, y=w835) -> (x-y=w826:dbl)
                                n371 = Greater Or Equal?(x=w827, y=w828) -> (x >= y?=w830:bool)
                                n372 = Greater Or Equal?(x=w828, y=w826) -> (x >= y?=w831:bool)
                                n373 = In Range and Coerce(upper limit=w827, x=w828, lower limit=w826) -> ()  [unwired: 2 out]
                                n374 = And(x=w830, y=w831) -> (x .and. y?=w829:bool)
                                }
                                n375 = case shown="真" w752 {
                                tunnel: w751 -> [_ w763]
                                frame False {
                                }
                                frame True {
                                w770 = ""
                                n376 = property on="多通道/单通道" class="Bool (严格)"() -> ("Value"=w757:bool)  [unwired: 2 in, 2 out]
                                n377 = property on="传感器顺序编号（从1开始）" class="Arr (严格)"() -> ("Value"=w761:string[])  [unwired: 2 in, 2 out]
                                n378 = property on="传感器顺序编号（从1开始）" class="Arr (严格)"() -> ("Value"=w773:string[])  [unwired: 2 in, 2 out]
                                n379 = Array Size(array=w761) -> (size(s)=w759:i32)
                                n380 = Array Size(array=w773) -> (size(s)=w778:i32)
                                n381 = Interleave 1D Arrays(w773, string[] [" ", " ", " ", " ", " ", " ", " ", " ", " ", " "]) -> (w771:string[])
                                n382 = Multiply(x=2, y=w778) -> (x*y=w760:i32)
                                n383 = case shown="真" w757 {
                                tunnel: w760 -> [w784 w793]
                                tunnel: w759 -> [_ w792]
                                tunnel: [w783 w791] -> w758
                                frame False {
                                w786 = u16 0 items=["DC Voltage", "AC Voltage", "2 - Wire Resistance", "4 - Wire Resistance", "DC Current", "AC Current", "Frequency", "Period", "Continuity", "Diode Checking", "VDC:VDC Ratio", "Temperature", "Capacitance"] ("Function (0: DC Voltage)")
                                n384 = property on="HP34401" class="VISAName"() -> ("Value"=w785:refnum<visa-resource-name>)  [unwired: 2 in, 2 out]
                                n385 = for {
                                N: w784 -> [_]
                                tunnel: w785 -> [w790]
                                tunnel: w786 -> [w789]
                                tunnel: [w787] -> w783 mode=indexing
                                n386 = call "Agilent 34401.vi"("Function (0: DC Voltage)"=w789, "VISA resource name"=w790) -> ("Measurement"=w788:dbl)  [unwired: 1 in, 1 out]
                                n387 = Number To Fractional String(number=w788) -> (F-format string=w787:string)  [unwired: 3 in]
                                }
                                }
                                frame True {
                                n388 = flat-sequence {
                                tunnel: w793 -> [w802]
                                tunnel: w792 -> [w801]
                                tunnel: [w800] -> w791
                                frame #0 {
                                n389 = property on="测试时断开电源？" class="Bool (严格)"() -> ("Value"=w794:bool)  [unwired: 2 in, 2 out]
                                n390 = case shown="真" w794 {
                                frame False {
                                }
                                frame True {
                                n391 = property on="控制板" class="VISAName"() -> ("Value"=w798:refnum<visa-resource-name>)  [unwired: 2 in, 2 out]
                                n392 = property on="传感器顺序编号（从1开始）" class="Arr (严格)"() -> ("Value"=w797:string[])  [unwired: 2 in, 2 out]
                                n393 = Array Size(array=w797) -> (size(s)=w796:i32)
                                n394 = call "prepare_elec_sensor.vi"("打开"=FALSE, "传感器数目"=w796, "VISA资源名称"=w798) -> ()  [unwired: 9 in]
                                }
                                }
                                }
                                frame #1 {
                                n395 = property on="测试时断开电源？" class="Bool (严格)"() -> ("Value"=w799:bool)  [unwired: 2 in, 2 out]
                                n396 = property on="组装调试" class="Bool (严格)"() -> ("Value"=w803:bool)  [unwired: 2 in, 2 out]
                                n397 = property on="控制板" class="VISAName"() -> ("Value"=w805:refnum<visa-resource-name>)  [unwired: 2 in, 2 out]
                                n398 = property on="HP34401" class="VISAName"() -> ("Value"=w804:refnum<visa-resource-name>)  [unwired: 2 in, 2 out]
                                n399 = case shown="真" w803 {
                                tunnel: [w807 w815] -> w800
                                tunnel: w804 -> [w811 w816]
                                tunnel: w802 -> [_ _]
                                tunnel: w801 -> [w809 w814]
                                tunnel: w805 -> [w810 w813]
                                tunnel: w799 -> [w806 w812]
                                frame False {
                                n400 = call "getMultiChannelsVoltage.vi"("测试时断开电源？"=w806, "调试？T/F"=FALSE, "传感器数目"=w809, "控制板"=w810, "电压表"=w811) -> ("获取结果"=w807:string[])  [unwired: 6 in]
                                }
                                frame True {
                                n401 = call "getMultiChannelsVoltage.vi"("测试时断开电源？"=w812, "传感器数目"=w814, "控制板"=w813, "电压表"=w816) -> ("获取结果"=w815:string[])  [unwired: 7 in]
                                }
                                }
                                }
                                frame #2 {
                                n402 = property on="测试时断开电源？" class="Bool (严格)"() -> ("Value"=w817:bool)  [unwired: 2 in, 2 out]
                                n403 = case shown="真" w817 {
                                frame False {
                                }
                                frame True {
                                (unwired) TRUE ("打开")
                                n404 = property on="控制板" class="VISAName"() -> ("Value"=w820:refnum<visa-resource-name>)  [unwired: 2 in, 2 out]
                                n405 = property on="传感器顺序编号（从1开始）" class="Arr (严格)"() -> ("Value"=w819:string[])  [unwired: 2 in, 2 out]
                                n406 = Array Size(array=w819) -> (size(s)=w818:i32)
                                n407 = call "prepare_elec_sensor.vi"("传感器数目"=w818, "VISA资源名称"=w820) -> ()  [unwired: 10 in]
                                }
                                }
                                }
                                }
                                }
                                }
                                n408 = Add(x=3, y=w760) -> (x+y=w774:i32)
                                n409 = Build Array (concatenate)(w770, w770, w770, w771) -> (w768:string[])
                                n410 = Array Subset(array=string[] ["时间", "温度（℃）", "压力（KPa）", "电压1（V）", "桥压1（V）", "电压2（V）", "桥压2（V）", "电压3（V）", "桥压3（V）", "电压4（V）", "桥压4（V）", "电压5（V）", "桥压5（V）", "电压6（V）", "桥压6（V）", "电压7（V)", "桥压7（V)", "电压8（V）", "桥压8（V）", "电压9（V)", "桥压9（V）", "电压10（V)", "桥压10（V）"], index=0 ("索引"), length=w774) -> (w769:string[])
                                n411 = disable-structure shown="禁用" {
                                frame Disabled {
                                w821 = u16 0 items=["DC Voltage", "AC Voltage", "2 - Wire Resistance", "4 - Wire Resistance", "DC Current", "AC Current", "Frequency", "Period", "Continuity", "Diode Checking", "VDC:VDC Ratio", "Temperature", "Capacitance"] ("Function (0: DC Voltage)")
                                n412 = for {
                                tunnel: _ -> [w825]
                                tunnel: w821 -> [w824]
                                tunnel: [w822] -> _ mode=indexing
                                n413 = call "Agilent 34401.vi"("Function (0: DC Voltage)"=w824, "VISA resource name"=w825) -> ("Measurement"=w823:dbl)  [unwired: 1 in, 1 out]
                                n414 = Number To Fractional String(number=w823) -> (F-format string=w822:string)  [unwired: 3 in]
                                }
                                }
                                frame Enabled {
                                }
                                }
                                n415 = Build Array(w769, w768) -> (w765:string[][])
                                n416 = Get Date/Time String(want seconds? (F)=TRUE ("disable buffering (T)")) -> (time string=w781:string)  [unwired: 2 in, 1 out]
                                n417 = property on="实时压力kPa" class="Str"() -> ("Value"=w779:string)  [unwired: 2 in, 2 out]
                                n418 = Number To Fractional String(number=w763) -> (F-format string=w780:string)  [unwired: 3 in]
                                n419 = property on="时漂常压输出" class="Arr (严格)"() -> ("Value"=w767:string[][])  [unwired: 2 in, 2 out]
                                n420 = Build Array (concatenate)(w781, w780, w779, w758) -> (w766:string[])
                                n421 = Build Array (concatenate)(w767, w766) -> (w764:string[][])
                                n422 = property on="时漂常压输出" class="Arr (严格)"("Value"=w764) -> ()  [unwired: 2 in, 2 out]
                                n423 = Insert Into Array(array=w765, new element=w764) -> (w762:string[][])  [unwired: 2 in]
                                n424 = property on="时漂测试数据" class="MCListbox (严格)"("ItemNames"=w762) -> ()  [unwired: 2 in, 2 out]
                                }
                                }
                                }
                                frame #6 {
                                n425 = property on="压力稳定" class="Bool (严格)"("Value"=FALSE ("压力稳定")) -> ()  [unwired: 2 in, 2 out]
                                }
                                frame #7 {
                                n426 = Less?(x=w838, y=8.0) -> (x < y?=w837:bool)
                                n427 = case shown="真" w837 {
                                frame False {
                                }
                                frame True {
                                n428 = property on="时漂测试间隔时间(min)" class="DigNum (严格)"() -> ("Value"=w842:i32)  [unwired: 2 in, 2 out]
                                n429 = Multiply(x=w842, y=60000) -> (x*y=w840:i32)
                                n430 = Wait Until Next ms Multiple(millisecond multiple=w840) -> ()  [unwired: 1 out]
                                }
                                }
                                }
                                }
                                }
                              }
                              frame #1 {
                                n431 = property on="开始采集" class="Bool (严格)"("Value"=FALSE ("开始采集")) -> ()  [unwired: 2 in, 2 out]
                                n432 = property on="压力稳定" class="Bool (严格)"("Value"=FALSE ("压力稳定")) -> ()  [unwired: 2 in, 2 out]
                                n433 = property on="结束" class="Bool (严格)"("Value"=TRUE ("结束")) -> ()  [unwired: 2 in, 2 out]
                              }
                            }
                          }
                        }
                        n434 = disable-structure shown="禁用" {
                          frame Disabled {
                            n435 = String To Path() -> ()  [unwired: 1 in, 1 out]
                          }
                          frame Enabled {
                          }
                        }
                        n436 = Not(x=w442) -> (.not. x?=w448:bool)
                        n437 = case shown="真" w448 {
                          frame False {
                          }
                          frame True {
                            # "不是时漂执行该序列"
                            n438 = property on="压力设定值（KPa）" class="Arr (严格)"() -> ("Value"=w486:dbl[])  [unwired: 2 in, 2 out]
                            n439 = property on="压力设定值（KPa）" class="Arr (严格)"() -> ("Value"=w492:dbl[])  [unwired: 2 in, 2 out]
                            n440 = Reverse 1D Array(array=w486) -> (reversed array=w488:dbl[])
                            n441 = Array Max & Min(array=w486) -> (max value=w483:dbl, min value=w484:dbl)  [unwired: 2 out]
                            n442 = property on="检定次数" class="DigNum (严格)"() -> ("Value"=w494:i32)  [unwired: 2 in, 2 out]
                            n443 = Sort 1D Array(array=w492) -> (sorted array=w491:dbl[])
                            n444 = Multiply(x=1.01, y=w483) -> (x*y=w487:dbl)
                            n445 = Multiply(x=w484, y=0.99) -> (x*y=w485:dbl)
                            n446 = property on="压力设定值（KPa）" class="Arr (严格)"("Value"=w491) -> ()  [unwired: 2 in, 2 out]
                            n447 = Array Size(array=w491) -> (size(s)=w497:i32)
                            n448 = Increment(x=w497) -> (x+1=w496:i32)
                            n449 = Build Array (concatenate)(w485, w486, w487, w488) -> (w479:dbl[])
                            n450 = Array Max & Min(array=w479) -> (max value=→"压力最大值":dbl, min value=→"压力最小值":dbl)  [unwired: 2 out]
                            n451 = Multiply(x=2, y=w496) -> (x*y=w493:i32)
                            n452 = Multiply(x=w493, y=w494) -> (x*y=w478:i32)
                            n453 = Array Size(array=w479) -> (size(s)=w480:i32)
                            n454 = flat-sequence {
                              tunnel: w479 -> [w500]
                              tunnel: w480 -> [w499]
                              tunnel: w478 -> [w498]
                              frame #0 {
                                n455 = for {
                                N: w498 -> [_]
                                tunnel: w500 -> [w518]
                                tunnel: w499 -> [w503]
                                i -> [w516]
                                # "执行序列"
                                n456 = Greater Or Equal?(x=w516, y=w503) -> (x >= y?=w517:bool)
                                n457 = case shown="真" w517 {
                                tunnel: w516 -> [w519 w522]
                                tunnel: w503 -> [_ w521]
                                tunnel: [w519 w520] -> w515
                                frame False {
                                }
                                frame True {
                                n458 = Quotient & Remainder(x=w522, y=w521) -> (x-y*floor(x/y)=w520:i32)  [unwired: 1 out]
                                }
                                }
                                n459 = Index Array(array=w518, index=w515) -> (element=w501:dbl)
                                n460 = flat-sequence {
                                tunnel: w501 -> [w525]
                                tunnel: [w524] -> w513
                                tunnel: [w523] -> w502
                                tunnel: [w529] -> w514
                                tunnel: w513 -> [w529]
                                tunnel: [w528] -> w512
                                tunnel: w502 -> [w528]
                                tunnel: w514 -> [w541]
                                tunnel: w512 -> [w540]
                                tunnel: [w538] -> w511
                                tunnel: [w537] -> w510
                                tunnel: [w536] -> w509
                                tunnel: w501 -> [w531]
                                tunnel: w511 -> [w550]
                                tunnel: w510 -> [w556]
                                tunnel: w509 -> [w555]
                                tunnel: w501 -> [w554]
                                tunnel: [w553] -> w508
                                tunnel: [w552] -> w507
                                tunnel: [w551] -> w506
                                tunnel: [w550] -> w504
                                tunnel: w508 -> [_]
                                tunnel: w507 -> [w590]
                                tunnel: w506 -> [w589]
                                tunnel: [w587] -> w505
                                tunnel: w504 -> [w587]
                                tunnel: w505 -> [w593]
                                frame #0 {
                                n461 = property on="CONST820" class="VISAName"() -> ("Value"=w526:refnum<visa-resource-name>)  [unwired: 2 in, 2 out]
                                n462 = call "设定压力.vi"("设定"=w525, "VISA resource name"=w526) -> ("错误输出"=w523:errorcluster, "VISA资源名称输出"=w524:refnum<visa-resource-name>)  [unwired: 1 in]
                                }
                                frame #1 {
                                n463 = Wait (ms)(milliseconds to wait=u32 100 ("毫秒计时值")) -> ()  [unwired: 1 out]
                                }
                                frame #2 {
                                n464 = property on="压力最大值" class="DigNum (严格)"() -> ("Value"=w532:dbl)  [unwired: 2 in, 2 out]
                                n465 = property on="压力最小值" class="DigNum (严格)"() -> ("Value"=w533:dbl)  [unwired: 2 in, 2 out]
                                n466 = while {
                                tunnel: w541 -> [w546]
                                tunnel: w540 -> [w545]
                                tunnel: [w548] -> w539
                                tunnel: [w544] -> w537
                                tunnel: [w543] -> w536
                                stop <- w548 stop-if-true
                                # "1稳定 0不稳定"
                                n467 = call "压力稳定状态.vi"("error in (no error) 2"=w545, "VISA resource name"=w546) -> ("错误输出"=w543:errorcluster, "状态(1稳定)"=w542:string, "VISA资源名称输出"=w544:refnum<visa-resource-name>)  [unwired: 1 in]
                                n468 = Wait Until Next ms Multiple(millisecond multiple=u32 10 ("毫秒倍数")) -> ()  [unwired: 1 out]
                                n469 = Decimal String To Number(string=w542) -> (number=w549:i32)  [unwired: 2 in, 1 out]
                                n470 = Greater Than 0?(x=w549) -> (x > 0?=w548:bool)
                                }
                                n471 = Equal?(x=w531, y=w532) -> (x = y?=w535:bool)
                                n472 = Equal?(x=w533, y=w531) -> (x = y?=w534:bool)
                                n473 = Not Or(1:w535, 2:w534) -> (0:w530:bool)
                                n474 = And(x=w530, y=w539) -> (x .and. y?=w538:bool)
                                n475 = property on="压力稳定" class="Bool (严格)"("Value"=w538) -> ()  [unwired: 2 in, 2 out]
                                }
                                frame #3 {
                                n476 = case shown="真" w550 {
                                tunnel: w556 -> [w558 w570]
                                tunnel: w555 -> [w557 w569]
                                tunnel: [w559 w568] -> w553
                                tunnel: w554 -> [w561 w567]
                                tunnel: [w558 w566] -> w552
                                tunnel: [w557 w565] -> w551
                                frame False {
                                n477 = property on="压力最小值" class="DigNum (严格)"() -> ("Value"=w562:dbl)  [unwired: 2 in, 2 out]
                                n478 = Equal?(x=w562, y=w561) -> (x = y?=w560:bool)
                                n479 = case shown="真" w560 {
                                tunnel: ["反行程" "正行程"] -> w559
                                frame False {
                                }
                                frame True {
                                }
                                }
                                }
                                frame True {
                                n480 = while {
                                tunnel: w570 -> [w578]
                                tunnel: w569 -> [w579]
                                tunnel: [w577] -> w566
                                tunnel: [w575] -> w565
                                tunnel: [w585] -> w568
                                tunnel: w567 -> [w583]
                                stop <- w581 stop-if-true
                                w573 = 1.0 ("上限")
                                n481 = call "CONST820目标压力测量.vi"("error in (no error) 2"=w579, "VISA resource name"=w578) -> ("错误输出"=w575:errorcluster, "目标压力值"=w576:string, "VISA资源名称输出"=w577:refnum<visa-resource-name>)  [unwired: 1 in]
                                n482 = property on="精度" class="DigNum (严格)"() -> ("Value"=w572:dbl)  [unwired: 2 in, 2 out]
                                n483 = Add(x=w573, y=w572) -> (x+y=w574:dbl)
                                n484 = Wait Until Next ms Multiple(millisecond multiple=u32 10 ("毫秒倍数")) -> ()  [unwired: 1 out]
                                n485 = Subtract(x=w573, y=w572) -> (x-y=w571:dbl)
                                n486 = Match Pattern(string=w576, regular expression="," ("正则表达式")) -> (before substring=w585:string)  [unwired: 1 in, 3 out]
                                n487 = property on="实时压力kPa" class="Str"("Value"=w585) -> ()  [unwired: 2 in, 2 out]
                                n488 = Fract/Exp String To Number(string=w585) -> (number=w584:dbl)  [unwired: 3 in, 1 out]
                                n489 = Divide(x=w584, y=w583) -> (x/y=w582:dbl)
                                n490 = In Range and Coerce(upper limit=w574, x=w582, lower limit=w571) -> (In Range?=w581:bool)  [unwired: 1 out]
                                }
                                }
                                }
                                }
                                frame #4 {
                                n491 = VISA Close(VISA resource name=w590, error in (no error)=w589) -> (error out=→"错误输出 2":errorcluster)
                                }
                                frame #5 {
                                # "可视化"
                                # "数据采集"
                                n492 = property on="当前设定温度℃" class="DigNum (严格)"() -> ("Value"=w597:dbl)  [unwired: 2 in, 2 out]
                                n493 = property on="GWS" class="VISAName"() -> (error out=w596:errorcluster, "Value"=w595:refnum<visa-resource-name>)  [unwired: 2 in, 1 out]
                                n494 = while {
                                tunnel: w595 -> [w606]
                                tunnel: w596 -> [w605]
                                tunnel: w597 -> [w604]
                                tunnel: [w598] -> w594
                                tunnel: [w602] -> w591
                                stop <- w598 stop-if-true
                                w607 = 0.1
                                # "再次判断温度设置"
                                n495 = call "get_temp.vi"("错误输入（无错误）"=w605, "VISA资源名称"=w606) -> ("实时温度"=w602:dbl)  [unwired: 7 in, 2 out]
                                n496 = property on="实时温度℃" class="DigNum (严格)"("Value"=w602) -> ()  [unwired: 2 in, 2 out]
                                n497 = Add(x=w604, y=w607) -> (x+y=w603:dbl)
                                n498 = Subtract(x=w604, y=w607) -> (x-y=w601:dbl)
                                n499 = Greater Or Equal?(x=w603, y=w602) -> (x >= y?=w599:bool)
                                n500 = Greater Or Equal?(x=w602, y=w601) -> (x >= y?=w600:bool)
                                n501 = In Range and Coerce(upper limit=w603, x=w602, lower limit=w601) -> ()  [unwired: 2 out]
                                n502 = And(x=w599, y=w600) -> (x .and. y?=w598:bool)
                                }
                                n503 = And(x=w593, y=w594) -> (x .and. y?=w592:bool)
                                n504 = case shown="真" w592 {
                                tunnel: w591 -> [_ w614]
                                frame False {
                                }
                                frame True {
                                w621 = ""
                                n505 = property on="多通道/单通道" class="Bool (严格)"() -> ("Value"=w608:bool)  [unwired: 2 in, 2 out]
                                n506 = property on="传感器顺序编号（从1开始）" class="Arr (严格)"() -> ("Value"=w612:string[])  [unwired: 2 in, 2 out]
                                n507 = property on="传感器顺序编号（从1开始）" class="Arr (严格)"() -> ("Value"=w624:string[])  [unwired: 2 in, 2 out]
                                n508 = Array Size(array=w612) -> (size(s)=w610:i32)
                                n509 = Array Size(array=w624) -> (size(s)=w630:i32)
                                n510 = Interleave 1D Arrays(w624, string[] [" ", " ", " ", " ", " ", " ", " ", " ", " ", " "]) -> (w622:string[])
                                n511 = Multiply(x=2, y=w630) -> (x*y=w611:i32)
                                n512 = case shown="真" w608 {
                                tunnel: w611 -> [w636 w645]
                                tunnel: w610 -> [_ w644]
                                tunnel: [w635 w643] -> w609
                                frame False {
                                w638 = u16 0 items=["DC Voltage", "AC Voltage", "2 - Wire Resistance", "4 - Wire Resistance", "DC Current", "AC Current", "Frequency", "Period", "Continuity", "Diode Checking", "VDC:VDC Ratio", "Temperature", "Capacitance"] ("Function (0: DC Voltage)")
                                n513 = property on="HP34401" class="VISAName"() -> ("Value"=w637:refnum<visa-resource-name>)  [unwired: 2 in, 2 out]
                                n514 = for {
                                N: w636 -> [_]
                                tunnel: w637 -> [w642]
                                tunnel: w638 -> [w641]
                                tunnel: [w639] -> w635 mode=indexing
                                n515 = call "Agilent 34401.vi"("Function (0: DC Voltage)"=w641, "VISA resource name"=w642) -> ("Measurement"=w640:dbl)  [unwired: 1 in, 1 out]
                                n516 = Number To Fractional String(number=w640) -> (F-format string=w639:string)  [unwired: 3 in]
                                }
                                }
                                frame True {
                                n517 = flat-sequence {
                                tunnel: w645 -> [w654]
                                tunnel: w644 -> [w653]
                                tunnel: [w652] -> w643
                                frame #0 {
                                n518 = property on="测试时断开电源？" class="Bool (严格)"() -> ("Value"=w646:bool)  [unwired: 2 in, 2 out]
                                n519 = case shown="真" w646 {
                                frame False {
                                }
                                frame True {
                                n520 = property on="控制板" class="VISAName"() -> ("Value"=w650:refnum<visa-resource-name>)  [unwired: 2 in, 2 out]
                                n521 = property on="传感器顺序编号（从1开始）" class="Arr (严格)"() -> ("Value"=w649:string[])  [unwired: 2 in, 2 out]
                                n522 = Array Size(array=w649) -> (size(s)=w648:i32)
                                n523 = call "prepare_elec_sensor.vi"("打开"=FALSE, "传感器数目"=w648, "VISA资源名称"=w650) -> ()  [unwired: 9 in]
                                }
                                }
                                }
                                frame #1 {
                                n524 = property on="组装调试" class="Bool (严格)"() -> ("Value"=w655:bool)  [unwired: 2 in, 2 out]
                                n525 = property on="控制板" class="VISAName"() -> ("Value"=w657:refnum<visa-resource-name>)  [unwired: 2 in, 2 out]
                                n526 = property on="HP34401" class="VISAName"() -> ("Value"=w656:refnum<visa-resource-name>)  [unwired: 2 in, 2 out]
                                n527 = property on="测试时断开电源？" class="Bool (严格)"() -> ("Value"=w651:bool)  [unwired: 2 in, 2 out]
                                n528 = case shown="真" w655 {
                                tunnel: [w659 w667] -> w652
                                tunnel: w656 -> [w663 w668]
                                tunnel: w654 -> [_ _]
                                tunnel: w653 -> [w661 w666]
                                tunnel: w657 -> [w662 w665]
                                tunnel: w651 -> [w658 w664]
                                frame False {
                                n529 = call "getMultiChannelsVoltage.vi"("测试时断开电源？"=w658, "调试？T/F"=FALSE, "传感器数目"=w661, "控制板"=w662, "电压表"=w663) -> ("获取结果"=w659:string[])  [unwired: 6 in]
                                }
                                frame True {
                                n530 = call "getMultiChannelsVoltage.vi"("测试时断开电源？"=w664, "传感器数目"=w666, "控制板"=w665, "电压表"=w668) -> ("获取结果"=w667:string[])  [unwired: 7 in]
                                }
                                }
                                }
                                frame #2 {
                                n531 = property on="测试时断开电源？" class="Bool (严格)"() -> ("Value"=w669:bool)  [unwired: 2 in, 2 out]
                                n532 = case shown="真" w669 {
                                frame False {
                                }
                                frame True {
                                n533 = property on="控制板" class="VISAName"() -> ("Value"=w673:refnum<visa-resource-name>)  [unwired: 2 in, 2 out]
                                n534 = property on="传感器顺序编号（从1开始）" class="Arr (严格)"() -> ("Value"=w672:string[])  [unwired: 2 in, 2 out]
                                n535 = Array Size(array=w672) -> (size(s)=w671:i32)
                                n536 = call "prepare_elec_sensor.vi"("打开"=TRUE, "传感器数目"=w671, "VISA资源名称"=w673) -> ()  [unwired: 9 in]
                                }
                                }
                                }
                                }
                                }
                                }
                                n537 = Add(x=3, y=w611) -> (x+y=w625:i32)
                                n538 = Build Array (concatenate)(w621, w621, w621, w622) -> (w619:string[])
                                n539 = Array Subset(array=string[] ["时间", "温度（℃）", "压力（KPa）", "电压1（V）", "桥压1（V）", "电压2（V）", "桥压2（V）", "电压3（V）", "桥压3（V）", "电压4（V）", "桥压4（V）", "电压5（V）", "桥压5（V）", "电压6（V）", "桥压6（V）", "电压7（V)", "桥压7（V)", "电压8（V）", "桥压8（V）", "电压9（V)", "桥压9（V）", "电压10（V)", "桥压10（V）"], index=0 ("索引"), length=w625) -> (w620:string[])
                                n540 = disable-structure shown="禁用" {
                                frame Disabled {
                                w674 = u16 0 items=["DC Voltage", "AC Voltage", "2 - Wire Resistance", "4 - Wire Resistance", "DC Current", "AC Current", "Frequency", "Period", "Continuity", "Diode Checking", "VDC:VDC Ratio", "Temperature", "Capacitance"] ("Function (0: DC Voltage)")
                                n541 = for {
                                tunnel: _ -> [w678]
                                tunnel: w674 -> [w677]
                                tunnel: [w675] -> _ mode=indexing
                                n542 = call "Agilent 34401.vi"("Function (0: DC Voltage)"=w677, "VISA resource name"=w678) -> ("Measurement"=w676:dbl)  [unwired: 1 in, 1 out]
                                n543 = Number To Fractional String(number=w676) -> (F-format string=w675:string)  [unwired: 3 in]
                                }
                                }
                                frame Enabled {
                                }
                                }
                                n544 = Build Array(w620, w619) -> (w616:string[][])
                                n545 = Get Date/Time String(want seconds? (F)=TRUE ("disable buffering (T)")) -> (time string=w633:string)  [unwired: 2 in, 1 out]
                                n546 = property on="实时压力kPa" class="Str"() -> ("Value"=w631:string)  [unwired: 2 in, 2 out]
                                n547 = Number To Fractional String(number=w614) -> (F-format string=w632:string)  [unwired: 3 in]
                                n548 = property on="数据" class="Arr (严格)"() -> ("Value"=w618:string[][])  [unwired: 2 in, 2 out]
                                n549 = Build Array (concatenate)(w633, w632, w631, w609) -> (w617:string[])
                                n550 = Build Array (concatenate)(w618, w617) -> (w615:string[][])
                                n551 = property on="数据" class="Arr (严格)"("Value"=w615) -> ()  [unwired: 2 in, 2 out]
                                n552 = Insert Into Array(array=w616, new element=w615) -> (w613:string[][])  [unwired: 2 in]
                                n553 = property on="显示数据" class="MCListbox (严格)"("ItemNames"=w613) -> ()  [unwired: 2 in, 2 out]
                                }
                                }
                                }
                                frame #6 {
                                n554 = property on="压力稳定" class="Bool (严格)"("Value"=FALSE ("压力稳定")) -> ()  [unwired: 2 in, 2 out]
                                }
                                }
                                }
                              }
                              frame #1 {
                                n555 = property on="开始采集" class="Bool (严格)"("Value"=FALSE ("开始采集")) -> ()  [unwired: 2 in, 2 out]
                                n556 = property on="压力稳定" class="Bool (严格)"("Value"=FALSE ("压力稳定")) -> ()  [unwired: 2 in, 2 out]
                                n557 = property on="结束" class="Bool (严格)"("Value"=TRUE ("结束")) -> ()  [unwired: 2 in, 2 out]
                              }
                            }
                          }
                        }
                      }
                    }
                  }
                  frame #6 {
                    # "关闭"
                    n558 = property on="结束" class="Bool (严格)"() -> ("Value"=w846:bool)  [unwired: 2 in, 2 out]
                    n559 = case shown="真" w846 {
                      frame False {
                      }
                      frame True {
                        w876 = "Measured Data"  # group name
                        # "恢复压力到常压"
                        # "结束"
                        # "数据保存"
                        n560 = property on="温度（℃）" class="Arr (严格)"() -> ("Value"=w875:dbl[])  [unwired: 2 in, 2 out]
                        n561 = property on="温度点" class="DigNum (严格)"() -> ("Value"=w874:i32)  [unwired: 2 in, 2 out]
                        n562 = property on="当前设定温度℃" class="DigNum (严格)"() -> ("Value"=w861:dbl)  [unwired: 2 in, 2 out]
                        n563 = property on="loging" class="Str"() -> ("Value"=w872:string)  [unwired: 2 in, 2 out]
                        n564 = Increment(x=w874) -> (x+1=w895:i32)
                        n565 = Index Array(array=w875, index=w874) -> ()  [unwired: 1 out]
                        n566 = Array Size(array=w875) -> (size(s)=w896:i32)
                        n567 = property on="温度校验次数" class="DigNum (严格)"("Value"=5.0 ("温度校验次数")) -> ()  [unwired: 2 in, 2 out]
                        n568 = Number To Fractional String(number=w861, precision (6)=i16 1 ("精度(6)")) -> (F-format string=w871:string)  [unwired: 2 in]
                        n569 = Concatenate Strings(w872, w871, "℃ " ("字符串"), "数据保存" ("字符串"), "\n") -> (w869:string)
                        n570 = property on="loging" class="Str"("Value"=w869) -> ()  [unwired: 2 in, 2 out]
                        n571 = Equal?(x=w895, y=w896) -> (x = y?=w865:bool)
                        n572 = case shown="真" w865 {
                          tunnel: w895 -> [w920 _]
                          tunnel: [w920 0] -> w894
                          frame False {
                          }
                          frame True {
                            w927 = u16 10 items=["1.0"=10, "1.5"=15, "2.0"=20] ("Serial Settings:Stop Bits")
                            w928 = u16 0 items=["None", "Odd", "Even", "Mark", "Space"] ("Serial Settings:Parity")
                            w926 = "\u000200014000.0000"
                            # "关闭电源"
                            n573 = property on="多通道/单通道" class="Bool (严格)"() -> ("Value"=w921:bool)  [unwired: 2 in, 2 out]
                            n574 = property on="GWS" class="VISAName"() -> ("Value"=w942:refnum<visa-resource-name>)  [unwired: 2 in, 2 out]
                            n575 = property on="DH1766-2" class="VISAName"() -> ("Value"=w932:refnum<visa-resource-name>)  [unwired: 2 in, 2 out]
                            n576 = case shown="真" w921 {
                              frame False {
                              }
                              frame True {
                                n577 = property on="控制板" class="VISAName"() -> ("Value"=w947:refnum<visa-resource-name>)  [unwired: 2 in, 2 out]
                                n578 = property on="传感器顺序编号（从1开始）" class="Arr (严格)"() -> ("Value"=w946:string[])  [unwired: 2 in, 2 out]
                                n579 = Array Size(array=w946) -> (size(s)=w945:i32)
                                n580 = call "prepare_elec_sensor.vi"("打开"=FALSE, "传感器数目"=w945, "VISA资源名称"=w947) -> ()  [unwired: 9 in]
                              }
                            }
                            n581 = call "CRC.vi"("命令字符串"=w926) -> ("校验字符串"=w933:string)  [unwired: 10 in]
                            n582 = Concatenate Strings(w926, w933, "\u0003" ("字符串")) -> (w936:string)
                            n583 = property class="Instr"(reference=w942, "Baud"=u32 19200 ("Serial Settings:Baud Rate"), "Data Bits"=u16 8 ("Serial Settings:Data Bits"), "Parity"=w928, "Stop Bits"=w927) -> (reference out=w939:refnum<visa-resource-name>)  [unwired: 1 in, 1 out]
                            n584 = call-poly "VISA Configure Serial Port"("VISA resource name"=w932, "Enable Termination\nChar (T)"=FALSE ("Enable Termination\nChar (T)"), "baud rate (9600)"=u32 9600) -> ("VISA resource name out"=w937:refnum<visa-resource-name>, "error out"=w938:errorcluster)  [unwired: 4 in, 7 out]
                            n585 = property on="START" class="Bool (严格)"("Value"=FALSE ("START")) -> ()  [unwired: 2 in, 2 out]
                            n586 = VISA Write(VISA resource name=w937, write buffer=w936, error in (no error)=w938) -> (VISA resource name out=w934:refnum<visa-resource-name>, error out=w935:errorcluster)  [unwired: 1 out]
                            n587 = VISA Write(VISA resource name=w939, write buffer="MODE,OFF" ("写入缓冲区")) -> (VISA resource name out=w941:refnum<visa-resource-name>, error out=w940:errorcluster)  [unwired: 1 in, 1 out]
                            n588 = VISA Close(VISA resource name=w934, error in (no error)=w935) -> ()  [unwired: 1 out]
                            n589 = VISA Close(VISA resource name=w941, error in (no error)=w940) -> ()  [unwired: 1 out]
                          }
                        }
                        n590 = property on="温度点" class="DigNum (严格)"("Value"=w894) -> ()  [unwired: 2 in, 2 out]
                        n591 = property on="结束" class="Bool (严格)"("Value"=FALSE ("结束")) -> ()  [unwired: 2 in, 2 out]
                        n592 = property on="时漂测试" class="Bool (严格)"() -> ("Value"=w863:bool)  [unwired: 2 in, 2 out]
                        n593 = property on="GWS" class="Bool (严格)"("Value"=FALSE ("GWS")) -> ()  [unwired: 2 in, 2 out]
                        n594 = case shown="假" w863 {
                          tunnel: [w917 w919] -> w864
                          frame False {
                            n595 = property on="数据" class="Arr (严格)"() -> ("Value"=w917:string[][])  [unwired: 2 in, 2 out]
                          }
                          frame True {
                            n596 = property on="时漂常压输出" class="Arr (严格)"() -> ("Value"=w919:string[][])  [unwired: 2 in, 2 out]
                            n597 = property on="时漂测试" class="Bool (严格)"("Value"=FALSE ("时漂测试")) -> ()  [unwired: 2 in, 2 out]
                          }
                        }
                        n598 = Transpose 2D Array(2D array=w864) -> (transposed array=w883:string[][])
                        n599 = Current VI's Path() -> (path=w862:path)
                        n600 = Strip Path(path=w862) -> (stripped path=w887:path)  [unwired: 1 out]
                        n601 = property on="path" class="Str"() -> ("Value"=w882:string)  [unwired: 2 in, 2 out]
                        n602 = disable-structure shown="禁用" {
                          frame Disabled {
                            # "不同温度下的满量程输出值"
                            n603 = property on="压力设定值（KPa）" class="Arr (严格)"() -> ("Value"=w904:dbl[])  [unwired: 2 in, 2 out]
                            n604 = Array Max & Min(array=w904) -> (max value=w903:dbl)  [unwired: 3 out]
                            n605 = Divide(x=w903, y=1000.0) -> (x/y=w902:dbl)
                            n606 = Multiply(x=w902) -> (y=w905:dbl, x*y=w901:dbl)
                          }
                          frame Enabled {
                          }
                        }
                        n607 = Build Path(base path=w887, name or relative path="data" ("字符串")) -> (appended path=w886:path)
                        n608 = property on="检定次数" class="DigNum (严格)"() -> ("Value"=w859:i32)  [unwired: 2 in, 2 out]
                        n609 = property on="压力设定值（KPa）" class="Arr (严格)"() -> ("Value"=w860:dbl[])  [unwired: 2 in, 2 out]
                        n610 = Build Path(base path=w886, name or relative path=w882) -> (appended path=w890:path)
                        n611 = property on="传感器显示编号" class="Ring (严格)"() -> ("Value"=w850:u16)  [unwired: 2 in, 2 out]
                        n612 = Array Size(array=w860) -> (size(s)=w858:i32)
                        n613 = Increment(x=w850) -> (x+1=w849:u16)
                        n614 = case shown="真" w863 {
                          tunnel: [w906 w909] -> w857
                          tunnel: w849 -> [_ w910]
                          frame False {
                            n615 = property on="数据" class="Arr (严格)"() -> ("Value"=w906:string[][])  [unwired: 2 in, 2 out]
                          }
                          frame True {
                            n616 = property on="时漂测试" class="Bool (严格)"("Value"=FALSE ("START")) -> ()  [unwired: 2 in, 2 out]
                            n617 = disable-structure shown="禁用" {
                              frame Disabled {
                                n618 = property on="温度（℃）" class="Arr (严格)"() -> ("Value"=w915:dbl[])  [unwired: 2 in, 2 out]
                                n619 = call "getNormalTempIndex.vi"("温度列表"=w915) -> ("常温索引"=w916:dbl)  [unwired: 10 in]
                                n620 = Index Array(index=w916) -> ()  [unwired: 1 in, 1 out]
                              }
                              frame Enabled {
                              }
                            }
                            n621 = property on="时漂常压输出" class="Arr (严格)"() -> ("Value"=w913:string[][])  [unwired: 2 in, 2 out]
                            n622 = call "getTimeMov.vi"("Yf·s"=4.6, "传感器索引"=w910, "不包含头的全量数组数据"=w913) -> ("时漂"=→"时漂":dbl)  [unwired: 8 in]
                            n623 = call "getDataFromTDMS.vi"("文件名称"="test") -> ("数据"=w909:string[][])  [unwired: 10 in]
                            n624 = property on="时漂测试" class="Bool (严格)"("Value"=FALSE ("时漂测试")) -> ()  [unwired: 2 in, 2 out]
                          }
                        }
                        n625 = TDMS Open(6:FALSE ("disable buffering (T)"), 7:enum16{"1.0", "2.0"}."2.0" ("file format version (2.0)"), 10:T2."open or create" ("operation"), 11:w890) -> (0:w888:errorcluster, 3:w885:refnum<k34>)  [unwired: 3 in]
                        n626 = call "getCluster.vi"("数据"=w857, "检定次数"=w859, "压力点个数"=w858, "传感器索引（1开始）"=w849) -> ("结果簇"=w847:cluster{dbl[], dbl[]}[], "曲线信息"=w855:string[])  [unwired: 4 in, 6 out]
                        n627 = property on="CONST820" class="VISAName"() -> ("Value"=w867:refnum<visa-resource-name>)  [unwired: 2 in, 2 out]
                        n628 = call "setConst820.vi"("VISA resource name"=w867, "输入命令"="output:MODE VENT") -> ("VISA资源名称输出"=w852:refnum<visa-resource-name>, "错误输出"=w851:errorcluster)  [unwired: 6 in, 1 out]
                        n629 = property on="XY图" class="XYGraph (严格)"("Value"=w847) -> ()  [unwired: 2 in, 2 out]
                        n630 = TDMS Write(0:w885, 1:enum16{"decimated", "interleaved"}."decimated" ("数据布局（0:降采样）"), 5:w876, 7:string[] ["时间", "温度（℃）", "压力（KPa）", "电压1（V）", "桥压1（V）", "电压2（V）", "桥压2（V）", "电压3（V）", "桥压3（V）", "电压4（V）", "桥压4（V）", "电压5（V）", "桥压5（V）", "电压6（V）", "桥压6（V）", "电压7（V)", "桥压7（V)", "电压8（V）", "桥压8（V）", "电压9（V)", "桥压9（V）", "电压10（V)", "桥压10（V）"], 9:w883, 11:w888) -> (4:w884:refnum<k34>, 15:w889:errorcluster)  [unwired: 2 out]
                        n631 = for {
                          tunnel: w855 -> [w897] mode=indexing
                          shift-right: [w899] -> w853
                          shift-left: "" -> [w898]
                          n632 = Concatenate Strings(w898, w897) -> (w899:string)
                        }
                        n633 = TDMS Close(8:w889, 11:w884) -> ()  [unwired: 2 out]
                        n634 = VISA Close(VISA resource name=w852, error in (no error)=w851) -> ()  [unwired: 1 out]
                        n635 = property on="曲线拟合参数" class="Str"("Value"=w853) -> ()  [unwired: 2 in, 2 out]
                      }
                    }
                  }
                }
              }
              frame True {
                n636 = String Length(string=w950) -> (length=w948:i32)
                n637 = Greater Than 0?(x=w948) -> (x > 0?=w949:bool)
                n638 = property on="START" class="Bool (严格)"("Value"=FALSE ("START")) -> ()  [unwired: 2 in, 2 out]
                n639 = case shown="真" w949 {
                  tunnel: w950 -> [_ w952]
                  frame False {
                  }
                  frame True {
                    n640 = call "显示对话框信息"("Message"=w952) -> ()  [unwired: 9 in, 2 out]
                  }
                }
              }
            }
          }
        }
      }
    }
  }
  n641 = while {
    stop <- FALSE stop-if-true
    n642 = event shown="[3] \"设备检查\": 值改变" {
      selector: _ -> [_ _ _ _ _ _]
      dyn-events: _ -> [_ _ _ _ _ _]
      timeout: _ -> [_ _ _ _ _ _]
      event Timeout {
        n643 = event-data() -> ()  [unwired: 1 in, 3 out]
      }
      event "STOP": Value Change {
        n644 = event-data() -> ()  [unwired: 1 in, 6 out]
        n645 = property on="STOP" class="Bool (严格)"() -> ("Value"=w955:bool)  [unwired: 2 in, 2 out]
        n646 = case shown="真" w955 {
          frame False {
          }
          frame True {
            w963 = u16 10 items=["1.0"=10, "1.5"=15, "2.0"=20] ("Serial Settings:Stop Bits")
            w964 = u16 0 items=["None", "Odd", "Even", "Mark", "Space"] ("Serial Settings:Parity")
            w962 = "\u000200014000.0000"
            w977 = FALSE ("START")
            # "关闭电源"
            n647 = property on="恒温开始" class="Bool (严格)"("Value"=w977) -> ()  [unwired: 2 in, 2 out]
            n648 = property on="传感器预热" class="Bool (严格)"("Value"=w977) -> ()  [unwired: 2 in, 2 out]
            n649 = property on="START" class="Bool (严格)"("Value"=w977) -> ()  [unwired: 2 in, 2 out]
            n650 = property on="GWS" class="Bool (严格)"("Value"=w977) -> ()  [unwired: 2 in, 2 out]
            n651 = property on="恒温中" class="Bool (严格)"("Value"=w977) -> ()  [unwired: 2 in, 2 out]
            n652 = property on="开始上电" class="Bool (严格)"("Value"=w977) -> ()  [unwired: 2 in, 2 out]
            n653 = property on="开始采集" class="Bool (严格)"("Value"=w977) -> ()  [unwired: 2 in, 2 out]
            n654 = property on="压力稳定" class="Bool (严格)"("Value"=w977) -> ()  [unwired: 2 in, 2 out]
            n655 = property on="GWS" class="VISAName"() -> ("Value"=w958:refnum<visa-resource-name>)  [unwired: 2 in, 2 out]
            n656 = property on="DH1766-2" class="VISAName"() -> ("Value"=w957:refnum<visa-resource-name>)  [unwired: 2 in, 2 out]
            n657 = property on="显示数据" class="MCListbox (严格)"("ItemNames"=string[][] []) -> ()  [unwired: 2 in, 2 out]
            n658 = call "CRC.vi"("命令字符串"=w962) -> ("校验字符串"=w976:string)  [unwired: 10 in]
            n659 = Concatenate Strings(w962, w976, "\u0003" ("字符串")) -> (w973:string)
            n660 = property class="Instr"(reference=w958, "Baud"=u32 19200 ("Serial Settings:Baud Rate"), "Data Bits"=u16 8 ("Serial Settings:Data Bits"), "Parity"=w964, "Stop Bits"=w963) -> (reference out=w970:refnum<visa-resource-name>)  [unwired: 1 in, 1 out]
            n661 = call-poly "VISA Configure Serial Port"("VISA resource name"=w957, "Enable Termination\nChar (T)"=FALSE ("Enable Termination\nChar (T)"), "baud rate (9600)"=u32 9600) -> ("VISA resource name out"=w972:refnum<visa-resource-name>, "error out"=w971:errorcluster)  [unwired: 4 in, 7 out]
            n662 = VISA Write(VISA resource name=w972, write buffer=w973, error in (no error)=w971) -> (VISA resource name out=w975:refnum<visa-resource-name>, error out=w974:errorcluster)  [unwired: 1 out]
            n663 = VISA Write(VISA resource name=w970, write buffer="MODE,OFF" ("写入缓冲区")) -> (VISA resource name out=w968:refnum<visa-resource-name>, error out=w969:errorcluster)  [unwired: 1 in, 1 out]
            n664 = VISA Close(VISA resource name=w975, error in (no error)=w974) -> ()  [unwired: 1 out]
            n665 = VISA Close(VISA resource name=w968, error in (no error)=w969) -> ()  [unwired: 1 out]
          }
        }
      }
      event "退出": Value Change {
        n666 = event-data() -> ("NewVal"=w978:bool)  [unwired: 1 in, 5 out]
        n667 = case shown="真" w978 {
          frame False {
          }
          frame True {
            n668 = flat-sequence {
              tunnel: [w982] -> w980
              frame #0 {
                n669 = property on="退出" class="Bool (严格)"("Value"=FALSE ("退出")) -> ()  [unwired: 2 in, 2 out]
              }
              frame #1 {
                n670 = control-ref of="本VI"() -> (w982:refnum<vi>)
              }
            }
            n671 = invoke class="VI" method="FP.Close"(reference=w980) -> (reference out=w979:refnum<vi>)  [unwired: 2 in, 2 out]
            n672 = invoke class="VI" method="Abort VI"(reference=w979) -> ()  [unwired: 2 in, 3 out]
          }
        }
      }
      event "设备检查": Value Change {
        n673 = event-data() -> ("NewVal"=w983:bool)  [unwired: 1 in, 5 out]
        n674 = case shown="真" w983 {
          frame False {
          }
          frame True {
            n675 = property on="设备检查" class="Bool (严格)"("Value"=FALSE ("设备检查")) -> ()  [unwired: 2 in, 2 out]
            n676 = Open VI Reference(vi path=path "equipment_debug.vi" ("VI路径")) -> (vi reference=w985:refnum<vi>)  [unwired: 5 in, 1 out]
            n677 = property class="VI"(reference=w985) -> (reference out=w986:refnum<vi>, "FP.State"=w989:T3)  [unwired: 1 in, 1 out]
            n678 = Equal?(x=T3."Closed", y=w989) -> (x = y?=w987:bool)
            n679 = case shown="真" w987 {
              tunnel: w986 -> [w991 w993]
              frame False {
                n680 = property class="VI"(reference=w991, "Front Panel.IsFrontmost"=TRUE ("前面板窗口:在最前")) -> ()  [unwired: 1 in, 2 out]
              }
              frame True {
                n681 = invoke class="VI" method="FP.Open"(reference=w993, "Activate"=TRUE ("激活？"), "State"=T3."Standard" ("状态")) -> (reference out=w996:refnum<vi>)  [unwired: 2 in, 4 out]
                n682 = invoke class="VI" method="Run VI"(reference=w996, "Wait until done"=FALSE ("结束前等待"), "Auto Dispose Ref"=TRUE ("自动销毁引用")) -> ()  [unwired: 2 in, 5 out]
              }
            }
          }
        }
      }
      event Panel Close {
        n683 = event-data() -> ()  [unwired: 1 in, 4 out]
        n684 = flat-sequence {
          tunnel: [w1001] -> w999
          frame #0 {
            n685 = property on="退出" class="Bool (严格)"("Value"=FALSE ("退出")) -> ()  [unwired: 2 in, 2 out]
          }
          frame #1 {
            n686 = control-ref of="本VI"() -> (w1001:refnum<vi>)
          }
        }
        n687 = invoke class="VI" method="Abort VI"(reference=w999) -> ()  [unwired: 2 in, 3 out]
      }
      event "时漂测试": Value Change {
        n688 = event-data() -> ()  [unwired: 1 in, 6 out]
        n689 = property on="时漂测试" class="Bool (严格)"() -> ("Value"=w1002:bool)  [unwired: 2 in, 2 out]
        n690 = case shown="真" w1002 {
          frame False {
          }
          frame True {
            n691 = property on="START" class="Bool (严格)"("Value"=TRUE ("START")) -> ()  [unwired: 2 in, 2 out]
          }
        }
      }
    }
  }
